vi "LIA Example Host_Backup.vi"() -> ()   [LabVIEW 2017]
uses:
  Program Files (x86)/National Instruments/LabVIEW 2017/examples/Lock-In Amplifier/lib/host/Public/pll settings.ctl
  Program Files (x86)/National Instruments/LabVIEW 2017/examples/Lock-In Amplifier/lib/host/Public/lock-in settings.ctl
  Program Files (x86)/National Instruments/LabVIEW 2017/examples/Lock-In Amplifier/lib/interface/Interface FPGA/LIA Host Interface FPGA.lvclass
  C:/Program Files (x86)/National Instruments/LabVIEW 2017/examples/Lock-In Amplifier/lib/interface/Interface/LIA Host Interface.lvclass
  Program Files (x86)/National Instruments/LabVIEW 2017/examples/Lock-In Amplifier/lib/host/Public/fpga type.ctl
  Program Files (x86)/National Instruments/LabVIEW 2017/examples/Lock-In Amplifier/lib/interface/Interface FPGA/Properties/FpgaSession_GET.vi
  <vilib>/Utility/error.llb/Error Cluster From Error Code.vi
  <vilib>/rvi/errors/niLvFpgaAdjustHostInterfaceError.vi
  <vilib>/rvi/interface/nirviReadWriteControl/nirviReadWriteControl.xnode
  Program Files (x86)/National Instruments/LabVIEW 2017/examples/Lock-In Amplifier/lib/interface/Interface/LIA Host Interface.lvclass
  Program Files (x86)/National Instruments/LabVIEW 2017/examples/Lock-In Amplifier/lib/host/Lock-In Amplifier Example Host.lvlib
  Program Files (x86)/National Instruments/LabVIEW 2017/examples/Lock-In Amplifier/lib/shared/Lock-In Amplifier Example Shared.lvlib
  NiFpgaLv.dll
  <vilib>/rvi/interface/Simulation/niFpgaSimulationCallBeginRW.vi
panel:
  out "pll.q 2":dbl format="%_48p"
  out "pll.vco output 0":fxp<+/-,49,1> format="%#_48g"
  in  "pll.digital config 1":T1={"highLevel"=0.25, "lowLevel"=0.0, "trigger slope"=enum."Positive"}
  in  "pll.digital config 0":T1={"highLevel"=0.25, "lowLevel"=0.0, "trigger slope"=enum."Positive"}
  out "VCO0":dbl[](graph)
  in  "Samples to Read":u32=8000
  out "Result 2":dbl[](graph)=[0.0039863680608536725, 0.0039834652267361085, 0.003976707928082593, 0.003972932599160282, 0.003975670154549236, 0.003979992004370958, 0.003981613977970053, 0.003982100791408192, 0.0039825360403185975, 0.003983392205484175, 0.003985155784781558, 0.003984236112244219, 0.0039802259708269574, 0.003977993518710993, 0.003977332793436194, 0.0039770510070652266, 0.003979204127283512, 0.003981587078878048, 0.003980760652855861, 0.0039774178100061746, 0.0039747546819085605, 0.003975039874942771, 0.003977747825071247, 0.0039813749933174415, 0.003983052660707128, 0.003981864532273667, 0.003980707623093961, 0.003980685672608732, 0.003980632950130394, 0.003980639859174508, 0.003981496097098532, 0.003981835448756967, 0.003981009233135141, 0.003980447530571761, 0.003980017903769632, 0.0039793657225813735, 0.003978886485345096, 0.003978374017005743, 0.003978338111379032, 0.003977708023223816, 0.003974879414400682, 0.0039745951340425896, 0.003978916724054073, 0.003980971523716979, 0.003979875685955788, 0.003980031947639625, 0.003978700378989306, 0.0039759508493841375, 0.003977706550082877, 0.003980981223845854, 0.003980924989904941, 0.00398142250305552, 0.003984342633570469, 0.003985365747847764, 0.003983618653697518, 0.003983156575361657, 0.003984289296932574, 0.003983852105562812, 0.003981528926592434, 0.003979874886696675, 0.003981149393075987, 0.003983128197289955, 0.003982228639004797, 0.003980362051087412, 0.0039805914885188655, 0.003982175398647137, 0.003983227587595888, 0.003982993287403955, 0.003983769026180169, 0.003986244327364255, 0.003986387282293714, 0.003983722992396274, 0.003980432940053473, 0.003977087834015251, 0.003975735503916292, 0.003977729861696195, 0.0039810309668320085, 0.003983694360997393, 0.003985280958577398, 0.003983765419355885, 0.0039787537520719635, 0.003976420955930517, 0.003979177981817055, 0.003980278551671726, 0.003979009157938231, 0.003980564610811761, 0.003982896997404296, 0.003982531965338463, 0.00398162174159325, 0.003981155296610277, 0.003979671906210392, 0.003977937452361379, 0.003976319041318493, 0.0039748268062937105, 0.003975209835147359, 0.0039775478932476726, 0.0039792342447318866, 0.0039792651251529506, 0.003979914577140006, 0.003981608970237078, 0.003981740884947264, 0.003979338128173823, 0.0039772901178909215, 0.003978316936557498, 0.003980306197649136, 0.00398038362175213, 0.003979091211200594, 0.003978807299668593, 0.0039803341878988565, 0.003981042283130753, 0.003979621539503979, 0.003978263643398434, 0.00397885543345211, 0.003980851549467365, 0.003981595814270996, 0.003979534090788055, 0.003976644021712945, 0.0039759454351617, 0.003977357538735612, 0.003978485334334718, 0.003978954978352067, 0.003979752948069682, 0.003980540928132936, 0.003980879798312971, 0.003980939042674783, 0.003981495778424931, 0.0039832350756685946, 0.003984854761938983, 0.003985806865545657, 0.003986168790386302, 0.003983807623814505, 0.003979934662757646, 0.0039786253007486495, 0.0039795163519576555, 0.003980124362455335, 0.0039801733132380475, 0.003981166017222749, 0.003982928364539291, 0.00398290963673646, 0.003980782033860497, 0.0039789779800912676, 0.00397887129554249, 0.003980306008061739, 0.003983353716844369, 0.0039864363131257565, 0.003987887348298469, 0.003988751753916426, 0.003988581162494825, 0.003985527563512181, 0.003981672344151345, 0.003980272419023447, 0.003979888466373754, 0.003978899040399707, 0.003978450628808996, 0.003978327225919375, 0.00397792878270558, 0.003977832419551143, 0.003977741498301615, 0.003977459137679066, 0.003979189237702964, 0.003982949173669057, 0.003983911545934435, 0.003982006472906676, 0.003982384069069882, 0.00398330875633608, 0.003980685479122946, 0.003977745299396019, 0.003978278723887712, 0.0039793920164360235, 0.003978522346022443, 0.003980289178526612, 0.003985997852957612, 0.003988900053516028, 0.003986682772698723, 0.0039831224667016924, 0.003981503976481135, 0.003983123018952358, 0.003985518575956754, 0.003985143703271976, 0.00398195098151325, 0.003980037191873144, 0.003981538653756876, 0.003981542610164564, 0.00397790470261859, 0.003975693240187895, 0.003978387944601431, 0.003982616675137925, 0.003983218136106197, 0.003982211133300878, 0.003982507056608711, 0.003982046262850494, 0.003981635628886928, 0.003982258332005895, 0.003981184985661619, 0.003980668172649484, 0.003984100761381162, 0.003986254732171504, 0.003983367253550932, 0.003980078001556476, 0.003980489638162108, 0.003984508043688629, 0.003988084422329789, 0.003986382148766199, 0.003981484856571877, 0.003978186889057839, 0.003977457434788827, 0.003979266253832761, 0.003982690198689834, 0.003984965342314285, 0.0039834752122414685, 0.003979459150927101, 0.003977443978254645, 0.003978120340943846, 0.003978689408389411, 0.003978751854910974, 0.003979787433988033, 0.003980742378349713, 0.003980678769189533, 0.003982001563511514, 0.003983002537985921, 0.003980921422917653, 0.003978639211764403, 0.0039771230758271735, 0.003976374483646863, 0.003976908953592146, 0.003977079620167436, 0.003977738506023549, 0.003978907819838595, 0.003978870881183955, 0.0039786991463899675, 0.003978616841237893, 0.003977851604700389, 0.003977172646033985, 0.003977513345587875, 0.003978066317637949, 0.00397721868815389, 0.00397542406202231, 0.003973658782307012, 0.00397292656829825, 0.003973899402993055, 0.00397513597871939, 0.003976900361861566, 0.003979478821891459, 0.003980359121710901, 0.0039797019576911785, 0.003979945313537775, 0.003982379006825405, 0.003986819454342757, 0.0039890652386413835, 0.003986060398149026, 0.0039831428691718225, 0.003984496901174192, 0.003986576065894574, 0.003986125938377407, 0.003983891985470712, 0.00398157511744908, 0.00397951127296237, 0.003978500593552686, 0.003979825058149692, 0.003981716302000313, 0.0039817107965979, 0.003980302784099287, 0.003980204028749741, 0.003983014364448184, 0.003984483776541842, 0.003981232134039498, 0.003978395893460694, 0.003978604787843064, 0.003978088591331617, 0.003977643745079901, 0.003981151958603502, 0.003986226271684498, 0.003986688539328525, 0.00398285040357346, 0.003980708004165844, 0.003981031427992134, 0.003980668626391776, 0.003979651616103598, 0.003978880317374354, 0.0039775128160220285, 0.003975690825220382, 0.003977410017621176, 0.003983342449600035, 0.003986190656399481, 0.003983476383350003, 0.003980341993989051, 0.003979157257465969, 0.003978985270725249, 0.003979413120663591, 0.003981198911517176, 0.003983381317756299, 0.003983605961403449, 0.0039822860156277055, 0.003980286417622783, 0.0039768475416357895, 0.0039736879869413134, 0.003972770043621574, 0.003972718526259669, 0.003974519130329869, 0.003978694161036032, 0.003981355840064537, 0.003981296759826837, 0.003979698372206024, 0.003977856657432809, 0.00397795431123421, 0.003979325723467235, 0.003979504894921478, 0.003979619472327822, 0.003981681112522701, 0.003983077441318316, 0.0039811273181025505, 0.003979710446469805, 0.003982873726931343, 0.003985895650077765, 0.003983582096489223, 0.003979810013697831, 0.00397870261963418, 0.003979241406293512, 0.0039797808985378245, 0.003978918139717365, 0.003977535777630392, 0.003977174279037845, 0.003976053026727283, 0.003974360610691553, 0.003975871192530825, 0.00398070376475112, 0.003983714770545892, 0.003981664143647305, 0.003978445706521472, 0.003977845953534627, 0.003977873227033018, 0.003977111770884702, 0.003976355870737198, 0.003975870071358403, 0.003976255642033605, 0.003977987642614486, 0.003980893140634532, 0.003983298672616521, 0.003982542737547836, 0.003980956373361125, 0.003981588316479783, 0.003981099924508738, 0.003979506507396805, 0.003980373061407154, 0.003981050034851546, 0.003979799943130195, 0.00398028280696532, 0.003982919770116164, 0.003984651620736739, 0.003984268351143069, 0.003981935069842658, 0.003979361748262011, 0.003979413820711289, 0.0039819091662637255, 0.003983965670700655, 0.003983195383880426, 0.003979696636904256, 0.003976488408046576, 0.003975787870275286, 0.003978753090618529, 0.003984324294290705, 0.003986722440874599, 0.003984446566004449, 0.003981566760577411, 0.003978855418056195, 0.003977232685187752, 0.003977853017734198, 0.003977827668488712, 0.003977424923808143, 0.0039797462142667165, 0.003983275621354706, 0.003984608790885146, 0.003984263274431654, 0.0039836428598223885, 0.003982289402402122, 0.00398261311929772, 0.003984805689974769, 0.00398377695311104, 0.003979480127359843, 0.003976828270854342, 0.0039763859903618175, 0.003975761395998334, 0.003976091456954722, 0.003979165513275957, 0.003982664353684002, 0.003982886581709554, 0.003980047955028987, 0.0039782590386969975, 0.003980073329210244, 0.003982235704850346, 0.003980773867120832, 0.003977555381209153, 0.003975791737709191, 0.003976838209866267, 0.003980355161348826, 0.003982344986444255, 0.003980347043544887, 0.0039783343900315375, 0.003979105245400305, 0.003979753856154792, 0.0039795020035409, 0.003980682978976577, 0.003983237818856397, 0.003984501894403985, 0.003981990599159561, 0.00397813845175732, 0.0039781783129500805, 0.003981379501095057, 0.003983800319659427, 0.0039857199195843344, 0.003987536828800084, 0.003987384995500621, 0.00398475975584641, 0.003981910972240386, 0.0039812156813270015, 0.003981220039018881, 0.0039801429716929786, 0.003979105844453436, 0.003979900872535141, 0.003981579430532582, 0.003981582347555906, 0.003980139039412083, 0.003978454091171029, 0.003976863715954396, 0.003976033921033562, 0.003977173694941979, 0.003980382420161796, 0.0039840586737615305, 0.0039858618097569475, 0.003984425281235036, 0.003983032946244676, 0.003984565855969025, 0.0039852864498371296, 0.003983009612780214, 0.003981139689177589, 0.0039812527004194544, 0.003981986646524029, 0.003982602846659465, 0.003983280589296684, 0.003983755474126229, 0.0039837132315740445, 0.0039846301134892, 0.003986989494256891, 0.003987488059080713, 0.003983309854404208, 0.0039782076721439665, 0.003976779404301029, 0.0039771905871550045, 0.003977556821407479, 0.003978054614384593, 0.003978322077760754, 0.0039783766773285115, 0.003978026682177368, 0.0039780700494545865, 0.003979334905626531, 0.003980275008436087, 0.003979583910159532, 0.00397806625697346, 0.003977480276853295, 0.003979673909992011, 0.003984152425644857, 0.003986619298023859, 0.003985231117281544, 0.003983500615001195, 0.0039827866633789085, 0.00398137160376901, 0.003980892041843191, 0.003983315682358909, 0.003984865480707667, 0.003983596493280533, 0.003981799731490589, 0.003979158738644041, 0.003977797917050028, 0.003979467394893473, 0.003980100236966837, 0.003979116334303563, 0.003979059817445155, 0.003979986584513668, 0.0039818453133389775, 0.003983893814555208, 0.00398348900651728, 0.003981362260961778, 0.003981989596956523, 0.0039837588119772446, 0.003981791127329015, 0.003979701420423474, 0.003981576725192654, 0.003983063143716834, 0.003982116890878562, 0.003982195467368155, 0.003982486462938863, 0.0039800567872538516, 0.003976082161468444, 0.003974055954040137, 0.003976633941831419, 0.003981412775821396, 0.003983640348413388, 0.003983357995347387, 0.003981415849163097, 0.003977919741453189, 0.003976384895548883, 0.003977484433454275, 0.003977252054023722, 0.0039765150670972235, 0.003978654275285551, 0.003981195762185493, 0.003981712475117914, 0.003981137882798154, 0.00397895360571178, 0.003975775432933715, 0.003975102135976764, 0.0039774497682601925, 0.003978427179725555, 0.003977365226889095, 0.003977594707952847, 0.0039767019639733135, 0.0039727506910756105, 0.0039727350006125706, 0.003978152009208106, 0.003980159374254768, 0.0039778710941888226, 0.003977375595577732, 0.003980037232534828, 0.003983264965478112, 0.003983324524760473, 0.003981049500959955, 0.003980003613294083, 0.003979577212737343, 0.003978403944249703, 0.003977237270009823, 0.003976316160817187, 0.003975980935475114, 0.003977003758017249, 0.003977453398748846, 0.003977510933683602, 0.00398058105512851, 0.0039848047947626366, 0.003986383499902778, 0.003985142716796781, 0.003983150027621312, 0.003983416133046983, 0.003985387313248186, 0.0039844723714048125, 0.003979539219264986, 0.003974621628978131, 0.003973281502577774, 0.0039751541913957454, 0.003977490665905324, 0.003979102054191885, 0.003979381596471701, 0.003977418001187858, 0.003974607390319347, 0.003972382924819207, 0.003971353084165621, 0.003972569948782476, 0.00397516451573597, 0.003976696824166696, 0.003977076730766446, 0.003978236385323944, 0.0039799412673816315, 0.003980671924222786, 0.003980012029596686, 0.003978637131431603, 0.003978993188237805, 0.0039814735245983805, 0.003982739573322356, 0.0039825759490366396, 0.003982518173980329, 0.003981344557208144, 0.003980092358437776, 0.0039806024039760555, 0.00398172681055136, 0.003982319799651587, 0.003981833044348206, 0.003980890395738155, 0.003980723786432255, 0.003980353748032666, 0.003979051107254107, 0.003978363950201649, 0.0039785129216881945, 0.003977883710210291, 0.003975881019731956, 0.003974052048585196, 0.003974685103243776, 0.003977958471936966, 0.003982240156118824, 0.003985098653442519, 0.003984012439980526, 0.003981088700704791, 0.0039804222812716275, 0.003981263262034946, 0.0039822816234043575, 0.003982610443778957, 0.003980656048561382, 0.00397770291899508, 0.003976242147367133, 0.003977345433387912, 0.003979314047879846, 0.003979744798891961, 0.003979349817858955, 0.003979659241239361, 0.0039804007065071135, 0.003980726381835716, 0.003981305356871311, 0.003983663642235815, 0.003987200737890198, 0.0039888053295015526, 0.003986669167392274, 0.003984745900617013, 0.003985989548151111, 0.0039860360759164885, 0.003982841996445306, 0.0039796657749838135, 0.003978478620282327, 0.003979000399240539, 0.003978465766836236, 0.003974640090741505, 0.003971365512208279, 0.003971996504204583, 0.003973775331863526, 0.003975569360546062, 0.003977651962298885, 0.003978271674510117, 0.003977967205246914, 0.00397737164455896, 0.003976686696863666, 0.0039777608428558245, 0.003979548577940783, 0.003980394891505464, 0.003981406684691207, 0.003981515105749858, 0.0039799934957620575, 0.003979236894441649, 0.003978711243243871, 0.003976779191494976, 0.003974763206625327, 0.003973968464875842, 0.003974932132657167, 0.0039789380515777685, 0.003984401295672218, 0.003986189522406129, 0.0039834701725929515, 0.003980876896964074, 0.003981219896273536, 0.00398161832558398, 0.003979026971481225, 0.0039764367788606364, 0.003976914121989127, 0.003978488293238594, 0.003979920584098437, 0.003981391784022643, 0.003981563759137481, 0.0039798070062099285, 0.003978446560805998, 0.003980264683577344, 0.0039827417583317495, 0.003982738530902676, 0.003981310720261693, 0.0039789152179851685, 0.003976986470379223, 0.003977691244145556, 0.0039782020428506416, 0.003976138976957626, 0.003975751526338582, 0.003978975755881895, 0.003981772145538809, 0.00398190266585997, 0.003980256210278689, 0.003978976266084329, 0.003979717924817937, 0.0039820618791054085, 0.003984055133639205, 0.0039842682843533785, 0.003983024743218702, 0.003980806628414367, 0.00397969919132365, 0.0039818567903902044, 0.003984262988199158, 0.003983554601450997, 0.003982491377327015, 0.0039842417870791244, 0.003985864763796289, 0.003984059717472494, 0.003979991963758913, 0.00397622112969835, 0.003975822545353304, 0.003978297051531639, 0.003979084757112439, 0.003979360358689138, 0.00398253720969874, 0.003984459419403273, 0.003981625031530332, 0.003977470787461008, 0.003975547484829462, 0.00397662570312401, 0.003979152537992211, 0.003981564827415988, 0.003983233356038698, 0.003982510000913845, 0.003980070544600705, 0.003977504202257701, 0.003975173437782767, 0.003975389538450331, 0.003977750496773989, 0.003979569013181202, 0.003981351513429408, 0.00398286798035896, 0.003982778257965616, 0.003980372431674904, 0.003976534269270507, 0.003976175306382319, 0.0039803233445810165, 0.00398337679753749, 0.0039834006955887895, 0.003983050335014145, 0.0039823805756204885, 0.003980064467056379, 0.003978699969180845, 0.003980115734287502, 0.003981333010629387, 0.003981386627589539, 0.003982395720148015, 0.003984079152264324, 0.003985038171922114, 0.003985167413950783, 0.003983941807828037, 0.003982038483599197, 0.003980884988355782, 0.003979008103024772, 0.003976990229437761, 0.003977162586203987, 0.003976899320749507, 0.003974284450258375, 0.0039720946084108285, 0.003972026230624667, 0.00397374886027822, 0.003976367439575529, 0.003977842425566234, 0.003977093338184401, 0.003976103952084634, 0.0039763017689312865, 0.003976092417151285, 0.003975060626111278, 0.003975065135869968, 0.0039763107365488526, 0.003977352867079649, 0.003977969349847659, 0.003978553095446936, 0.003979036478021424, 0.003978983042730239, 0.003978741465652077, 0.003979340578042503, 0.003979701242850902, 0.003978430882799382, 0.003976652233153723, 0.0039765179596725, 0.00397795735513347, 0.003979565201195335, 0.003981345484242718, 0.003981469312432307, 0.003978889562823616, 0.003976624913683742, 0.0039761610778784534, 0.003977824959453653, 0.00398214069195037, 0.00398742195165944, 0.0039896995458981776, 0.003986037631195687, 0.003979967695862646, 0.003977040393717214, 0.003977674391227534, 0.0039792757272066395, 0.003979552641289948, 0.003978935698737408, 0.003978281367870273, 0.003977642996036234, 0.003978731377392299, 0.003981539171295274, 0.003984238656581007, 0.003985224180818125, 0.003983057443176566, 0.003979499397401518, 0.003978410752375987, 0.003979776671656836, 0.003980391436479124, 0.003980049271568817, 0.003980241632899643, 0.003980339940009103, 0.0039807557540897055, 0.0039822609635872695, 0.003983176627180919, 0.003983926928775935, 0.003985551548307111, 0.003985646813215484, 0.003983680363220629, 0.003982849003454181, 0.003985561835201112, 0.003988929187930998, 0.003987829703049252, 0.003983503133059348, 0.003980623127040725, 0.003981481278276747, 0.003984305894978182, 0.003983197724472904, 0.003977985889312162, 0.003974146671127731, 0.003972623406271078, 0.0039726346931309026, 0.003974042725941328, 0.003976747169016437, 0.003981487948263495, 0.00398504490845982, 0.003983113583811858, 0.003978458043433113, 0.003976326104421417, 0.003977793620755946, 0.003980780035179106, 0.003981852492902647, 0.0039806181319497844, 0.003979685704064992, 0.0039783801316026325, 0.003976448851123849, 0.003976660341366401, 0.003978477345490919, 0.003980078187884992, 0.0039818262398588124, 0.003983429147918595, 0.003984344934371185, 0.00398413317542814, 0.003982099362293185, 0.003979385893110493, 0.00397997889618068, 0.0039846267580415816, 0.0039861289961856386, 0.003981209101616648, 0.003976602731196693, 0.003975722568327848, 0.0039750119685239855, 0.003974583143683917, 0.003977236560717556, 0.003982154517706716, 0.003986351620900945, 0.0039867699783994685, 0.003983698012302503, 0.003979936072057596, 0.003977518007059206, 0.003977251859838127, 0.003977404443913313, 0.003977064129850515, 0.0039774177115842945, 0.003978840238485831, 0.003981328955739816, 0.003983214287842484, 0.003982316329195417, 0.003979705808360979, 0.003978095353210538, 0.0039780303866684755, 0.003977773027807622, 0.003976670088152897, 0.0039760803031386625, 0.003977074375590223, 0.0039785954201575924, 0.00397900504669715, 0.003978684455654764, 0.003979150345052722, 0.003980073213741131, 0.00397922400508169, 0.003976634199148333, 0.003973792948548973, 0.003971947735484429, 0.003973449300176407, 0.003977365527006807, 0.003979173865527555, 0.003978565338237246, 0.003979438592656055, 0.003982226081643567, 0.003984568899889969, 0.003985383545762023, 0.00398379361244337, 0.003980766058359194, 0.0039789937389582706, 0.003978725628367393, 0.003978486455318838, 0.00397930624856685, 0.003983076144599588, 0.003986916500922116, 0.003987391456195043, 0.003985187981902368, 0.0039814220323227505, 0.0039782599038656885, 0.0039793530195430405, 0.0039836665900997974, 0.003985418628529121, 0.003983107447318631, 0.0039807533716833795, 0.003980452673891609, 0.00398121246321292, 0.003981579245847072, 0.0039806453902812115, 0.0039793147147476815, 0.003977426450764091, 0.003974647202875613, 0.003975534272025265, 0.003980944354864695, 0.0039837113287362075, 0.00398066195437423, 0.003976075275215913, 0.003973624263519756, 0.003972642118978977, 0.0039721981348636755, 0.003972418027957137, 0.003973516751950605, 0.003975424914188026, 0.0039764420265992395, 0.003976805487305147, 0.003977527309148269, 0.003977276759045344, 0.003977874650012254, 0.003981908131747179, 0.003985791593126928, 0.003987332531377609, 0.003988917999303813, 0.0039898000436693675, 0.003988775524159052, 0.003986804137343182, 0.003983974012608901, 0.003981762439486124, 0.0039812892508868285, 0.003981024159819735, 0.0039812211576087195, 0.00398236019474162, 0.003983547327636211, 0.003984231855020959, 0.003982225962846631, 0.0039783147688324414, 0.003977077736042259, 0.0039784658388757775, 0.003979775888746237, 0.003979987933157361, 0.003979458851215214, 0.0039793476299291725, 0.003978612550414, 0.003976314387840179, 0.003975056548604429, 0.003977366661085867, 0.003981128734793488, 0.003982649122544232, 0.003982768691437142, 0.003982005871057322, 0.003980190872963164, 0.0039813036494263454, 0.003984124532118742, 0.003982475946791014, 0.003977761415616033, 0.003974659343488677, 0.003972846843811938, 0.003972806715625865, 0.003975651569164522, 0.003977963611383471, 0.003977873468104301, 0.003978068385375542, 0.003979488335530391, 0.003979110480443132, 0.003977206961489088, 0.0039789202289513695, 0.003983288863755289, 0.003984077121378504, 0.0039822076981657125, 0.003981856479113935, 0.00398181012214159, 0.003980737648898447, 0.003980066845379656, 0.003978715861692618, 0.0039758546373015995, 0.003975257761946412, 0.003977846923118978, 0.003980669832971535, 0.003982954669011326, 0.0039835557510074, 0.003981614603206939, 0.003980593956608991, 0.0039822666237705985, 0.003982790656945957, 0.00398006863105295, 0.003977102352752207, 0.003976331524483975, 0.003976025112422648, 0.003975993713770331, 0.003978360261045454, 0.003980515957965241, 0.003980492262176662, 0.0039803134217181214, 0.003981116190908811, 0.003983517947269706, 0.003984911931008131, 0.0039824874179596684, 0.003979324028877534, 0.003976903166459353, 0.003973952933671413, 0.003972768156739406, 0.003974518699813129, 0.003977092525553969, 0.003979000361980179, 0.003979473587682066, 0.00397880296134308, 0.0039773501151807765, 0.003975775190348078, 0.003976784857872222, 0.003980497553940501, 0.003982816679431947, 0.003982101922554104, 0.00398090377027712, 0.003980526960595199, 0.003980273848589513, 0.00398004016560462, 0.0039796316262196724, 0.003978590884515269, 0.003977695523808001, 0.003978113283674883, 0.003978093677450509, 0.003976234690895188, 0.003975571953397801, 0.003977429275899129, 0.003979690179076107, 0.003981314699049087, 0.003982365023104846, 0.00398219328738418, 0.003979413083539485, 0.003976093378332462, 0.003977107605273904, 0.003981169964969415, 0.003983559556918537, 0.003983587714059575, 0.003981431842795316, 0.003978969249534734, 0.003978935715453941, 0.003980895947219992, 0.003982877361418654, 0.003982597564966746, 0.003980748884707083, 0.003980175712387027, 0.003981130286463459, 0.003980398082433253, 0.003977314767296546, 0.003978106092339979, 0.003983020800341056, 0.003984163473727247, 0.003981822309170868, 0.00398186832723127, 0.003983498351935705, 0.003982833932537083, 0.00397963340189174, 0.003976943389420637, 0.003977245664763129, 0.003979882345903582, 0.003982544930166112, 0.003982603116630313, 0.003980387169699541, 0.003978424228600121, 0.003976559770536161, 0.003975981643434425, 0.003978714956440631, 0.0039812885056061615, 0.003980169419182908, 0.003978061693649715, 0.003979346532064259, 0.0039829775933541214, 0.003983549530300931, 0.003980744676411625, 0.003979164800276976, 0.003980084512057897, 0.003981743527813305, 0.003982186814042334, 0.003981262059743135, 0.003980155795563241, 0.0039791162400227426, 0.003978750075723301, 0.003979895399989306, 0.003982175444757632, 0.0039839269838620696, 0.003982767707209037, 0.003979702364871831, 0.0039794049219338224, 0.0039808389302070256, 0.003979538938519838, 0.003977892739263718, 0.0039786753680560085, 0.003979574852086779, 0.003979358746771128, 0.003978307718653613, 0.003977615907680387, 0.003980297680133449, 0.00398455438897639, 0.003985124482927759, 0.0039830989248438795, 0.0039821580726706815, 0.003983029891208001, 0.003985361124408492, 0.003986676078649965, 0.003985371613000642, 0.003984264122271375, 0.003985115332201757, 0.003985380850084425, 0.003984091577875379, 0.00398348442375365, 0.003982335908804991, 0.003979130290729062, 0.0039765271382101374, 0.003975761283694023, 0.003977309789773401, 0.003980495824565586, 0.003982011694418642, 0.003982418786917205, 0.003983446588687851, 0.003983373050037224, 0.003981312358611243, 0.003979194733814413, 0.003978205677460493, 0.0039771896308695015, 0.0039760863754637644, 0.0039754517556096595, 0.003975021126421098, 0.0039743248319844705, 0.003974288300301103, 0.003976760901184927, 0.003978623824061758, 0.003977594513440992, 0.003978555080478624, 0.0039821930546257, 0.003983594593330003, 0.003982405089531026, 0.003981856594388102, 0.003982187387509669, 0.003981223313549715, 0.0039807403298629356, 0.003983347548875419, 0.00398522027841444, 0.003983423163518952, 0.003980738682966747, 0.003979015525778642, 0.00397895173097921, 0.0039793029748609295, 0.003977636235713472, 0.0039759450751720654, 0.003976485471559254, 0.003977655809397979, 0.003977429349678956, 0.003977993254621377, 0.003981879567469959, 0.003985239298407153, 0.003983416989748803, 0.003979679076637758, 0.003980365788350991, 0.00398253381694978, 0.003981285993316625, 0.003979848440676178, 0.003980921832108509, 0.003982172952809117, 0.003981158711881339, 0.0039800950644021515, 0.00398118948495695, 0.0039812176124992054, 0.003979616502188085, 0.003979039178311631, 0.003977916218000592, 0.003975378585060592, 0.003973131227205391, 0.003971918687654648, 0.0039734481724517925, 0.003976717516063116, 0.003977014875929817, 0.003973625298260909, 0.00397052208057938, 0.003971026897799082, 0.00397378807698498, 0.003973657752896502, 0.003971306556533753, 0.003973085672003789, 0.0039772575872008996, 0.003979194823547542, 0.003980317158812024, 0.003981292049856421, 0.0039831232472903105, 0.003987251711291331, 0.003989738525540101, 0.003987456983345958, 0.003984035239048443, 0.003981801724854245, 0.003979640732521801, 0.003978737305790658, 0.0039786476741947826, 0.00397791462118473, 0.0039777749317880026, 0.003978196073117516, 0.003978760709114377, 0.003979171876865028, 0.00397890829124455, 0.003979693827835825, 0.003982373595558498, 0.003984460873171954, 0.003983641771434025, 0.003980399820629003, 0.003977143685017755, 0.003976739331852892, 0.003978646828280886, 0.003979812280227829, 0.003981210448487633, 0.003983015756720717, 0.0039817333859492165, 0.003979002376219683, 0.003979107817471822, 0.003981211465274229, 0.003982606424709189, 0.0039832693787421585, 0.003983051654033211, 0.003979894748497823, 0.003975385528241426, 0.003973522960580348, 0.003974656401160778, 0.003978349370676319, 0.003982892688988913, 0.003983594701533446, 0.003981272021551873, 0.00398141035625862, 0.003984034138904719, 0.003986270231203048, 0.003987371878162886, 0.003985805363107296, 0.0039817409828335005, 0.0039800045857511165, 0.003982567734983381, 0.003985107690832858, 0.003984026682255706, 0.003981247498766315, 0.003979945374079749, 0.0039792207502099, 0.0039776515097977305, 0.003977553621094195, 0.003979640591280083, 0.003979802663149316, 0.003977016451329748, 0.003975536826100867, 0.0039779635670275015, 0.0039826413914955915, 0.003984064601877063, 0.003980053006106213, 0.003976825452021229, 0.003978578253056492, 0.003981962351984016, 0.003982619824916695, 0.003981592297708066, 0.003982013868026151, 0.003982298477104434, 0.003980510565228737, 0.003977882740497247, 0.003975967656348129, 0.003974813724179058, 0.00397367248316158, 0.003973745754006388, 0.0039765977484971975, 0.0039808396448549836, 0.003983537135687354, 0.003982979750045097, 0.0039799912584952395, 0.003977658737727139, 0.003977733078746502, 0.003978891204631039, 0.003979577122098112, 0.003978841805351333, 0.003976426768058204, 0.003974922818355137, 0.003977647373739251, 0.003981615548013295, 0.003980917845452167, 0.003977078549640621, 0.00397536837004931, 0.0039759780432128385, 0.0039762392964120645, 0.003976725341889077, 0.003978542997694838, 0.003979204759203014, 0.003978218625753375, 0.003978442388650503, 0.0039788453982813115, 0.003977975565517368, 0.003980073457269644, 0.003984761099604855, 0.003984821629434982, 0.003979963390238673, 0.003976945779116363, 0.003978204691117046, 0.003979426407224877, 0.003978475158178936, 0.003978531771511002, 0.003979999568456761, 0.003980753652738751, 0.003982165401077395, 0.003984447066973862, 0.003984125648018166, 0.003981421270245027, 0.003980137096143932, 0.003981451103728136, 0.003982679633245892, 0.003982258706786912, 0.003981488736817787, 0.003980199736889629, 0.003979185774484476, 0.003980638280255229, 0.003983363518089745, 0.003983860950202896, 0.003981813894202404, 0.00398042291412263, 0.003979831315147897, 0.003979837933985523, 0.003981936562422305, 0.003983040777982667, 0.00398078405540393, 0.003978119547563092, 0.003977041795773243, 0.003977311074221384, 0.003978894939935517, 0.003981016940009896, 0.003981602804992968, 0.003980790460175742, 0.003980832038069681, 0.003980246643918975, 0.0039769227718498, 0.003974138089899075, 0.003975488971503561, 0.003979858248285364, 0.003982834257554093, 0.003982224164074203, 0.003980711646259053, 0.003980044834544112, 0.003980217296298432, 0.0039817160981850605, 0.003983443484275833, 0.00398371428718893, 0.003982610604973739, 0.003981524871862345, 0.003980620390250896, 0.003980108148874865, 0.003980783373574936, 0.003982060412047107, 0.003983948662640071, 0.003986074427056052, 0.0039863962532675, 0.003985134297653663, 0.003985193406920106, 0.003985882297205966, 0.00398405309546629, 0.003982542021274245, 0.003983904862923795, 0.003983049463213574, 0.003978382592098956, 0.003975436268357411, 0.003976550738406553, 0.003978588341625853, 0.003978228638552719, 0.003976405440297321, 0.003976619742890873, 0.003978250186032161, 0.003978039025728405, 0.003977476248553813, 0.003979160885704842, 0.003981493321230651, 0.003982737572559862, 0.003982199226558208, 0.0039800803582359014, 0.003978621713377863, 0.0039789827585751045, 0.003980856722724818, 0.003982756548377972, 0.003982152493373126, 0.003980001403718744, 0.003977809718787921, 0.003974775668880134, 0.003972822966618998, 0.003974116674563762, 0.0039774266158550745, 0.00398013621130506, 0.0039805969751882725, 0.003980839984234072, 0.003981913158604893, 0.0039809020006479, 0.003978043639507173, 0.0039761023336582525, 0.003975735479197253, 0.003977237164066012, 0.003979156890400347, 0.003977959631900995, 0.003975664541786072, 0.003977015948163484, 0.003979800747511443, 0.00398036358261194, 0.0039791333003214744, 0.003977584037880255, 0.003977903249913146, 0.003980824679784317, 0.003982139767034596, 0.003979923660558457, 0.003979679130910815, 0.003982887698775242, 0.0039839573368327, 0.003981415865620109, 0.003980026959041138, 0.0039826530815789355, 0.003985032531173712, 0.003983170211885002, 0.003981229208051504, 0.0039831419107672975, 0.003985314929199347, 0.003984736539562992, 0.003982047625534495, 0.003978092253258514, 0.003976171860381736, 0.003977097600080971, 0.003976715465265732, 0.003975528628593147, 0.003976225728987328, 0.003976577835919223, 0.003976080688442137, 0.003977065463732254, 0.003979095970022937, 0.003980869775893732, 0.003980031320668816, 0.003976488044518928, 0.003976033855949846, 0.003980667305431748, 0.0039852116356552105, 0.0039850375694942325, 0.003981444890417225, 0.003979055176481802, 0.003979334454276697, 0.003981964690537828, 0.003985277726719733, 0.003985372395858868, 0.0039828274764985615, 0.00398149899661329, 0.003982572698372539, 0.003983587744335812, 0.0039811751383610535, 0.003978667166125552, 0.0039799350381902725, 0.003980131396301726, 0.00397701659831602, 0.003976251438084941, 0.003980000546690863, 0.003984326491579235, 0.003985406726219048, 0.0039823257385474325, 0.003978328034980272, 0.0039781141261135775, 0.0039825817773765605, 0.003987019086670008, 0.003986378504586017, 0.003982321435581621, 0.003979287104622096, 0.003978757690781972, 0.003979867479212055, 0.003980990323479186, 0.003981524507956091, 0.003980930294299735, 0.003979714774223713, 0.0039798609378699, 0.003980489633458653, 0.003980954515594047, 0.003982451454848569, 0.003983592354646729, 0.003983023643667566, 0.003981780453426345, 0.003980150677261656, 0.003977939858915903, 0.003976663953581718, 0.003976567267764581, 0.003976742276555209, 0.003977026113949605, 0.0039759017010204374, 0.003974620894287012, 0.003976550878632898, 0.0039794254344922226, 0.003980053670982793, 0.003978893617156679, 0.003976881683576605, 0.00397681165987789, 0.003980650125893448, 0.0039839316298084905, 0.003981472200463117, 0.0039760224680521015, 0.0039749080711558235, 0.003978573498169757, 0.003980834012888352, 0.003980277146134611, 0.0039798290866767646, 0.003979696358708986, 0.003979243706929482, 0.003979458656012906, 0.003980735616066876, 0.003981573829207304, 0.003981333949018392, 0.003980334275621537, 0.003979296577206264, 0.00398092191490291, 0.003984615251211943, 0.003986054489476058, 0.003984084777022521, 0.003980669260339174, 0.003977687646522303, 0.00397633130425075, 0.003976487048231085, 0.003975980482120383, 0.00397444740535783, 0.003974517679956067, 0.003976443223808739, 0.003978538570867421, 0.003978807200209765, 0.003977011707770822, 0.003976664972314686, 0.003978300482415657, 0.003979540018477265, 0.003980498057458205, 0.0039823678050551255, 0.00398426523072378, 0.0039835282605164635, 0.003981308831879845, 0.0039816179762867, 0.0039839099042353575, 0.003986082753664326, 0.003988042873930375, 0.003987392251139272, 0.0039838210259798895, 0.00398181843022356, 0.003983219826813076, 0.00398609138070574, 0.003986520539064208, 0.003982348342074492, 0.003977350315412907, 0.003974825714130103, 0.003975001827794674, 0.003977881508835268, 0.00397983876716173, 0.003978133890651639, 0.003976987943834461, 0.003979209753329046, 0.003981358977343799, 0.0039804571205447345, 0.003978705675329452, 0.0039804624250637495, 0.0039837235542263625, 0.003982785445988357, 0.003979053783229923, 0.003977419940931196, 0.003979800732348097, 0.003984036663505942, 0.003984974435885952, 0.003981722544176443, 0.003978600948416513, 0.003978002716351739, 0.003978319099118849, 0.003977869650191021, 0.003977770879884532, 0.003979235856318206, 0.003980787554768288, 0.003981054721549102, 0.003981475992411021, 0.003983322700911616, 0.00398459773304639, 0.003983058390335627, 0.0039794076200789594, 0.003977001169472031, 0.00397933347944537, 0.0039834383415941034, 0.003981871562804738, 0.003976686265121069, 0.003976457926069695, 0.003980452398060831, 0.003982842756804102, 0.003983116591155044, 0.003983704020879471, 0.003986445190217968, 0.00398909119912337, 0.003987010336441944, 0.003983414412622325, 0.003984104843046473, 0.00398551784454822, 0.003983372321284873, 0.00398108339487192, 0.003981720491102667, 0.00398191641173596, 0.003978647712721205, 0.003975995437829183, 0.003977792287636826, 0.003980350600781975, 0.003980040640280543, 0.00397852709799242, 0.003976632207578901, 0.0039753732216189636, 0.003976682038481194, 0.003978276072790252, 0.003979894658056205, 0.003982765760135251, 0.003983833023602612, 0.003981797166506561, 0.00397954894130544, 0.003980166421746046, 0.00398235147254963, 0.003982998746410941, 0.0039811285591011755, 0.003977696908878916, 0.003977118739538499, 0.00398008944064117, 0.003981482740950911, 0.003979930882977621, 0.00397743087136605, 0.003975971252553409, 0.003977462863057397, 0.003980674791534549, 0.003982380782257275, 0.003981526409016917, 0.003980107334962722, 0.003981167294126887, 0.003983703414652771, 0.00398420490645264, 0.003982791413991762, 0.003981005836849114, 0.003978678257854902, 0.003976499847155555, 0.003977437797218255, 0.003980424883737011, 0.003980326027344289, 0.003979196440516551, 0.003980845589105199, 0.003981763032187864, 0.003981054495160551, 0.003981235591409589, 0.003980451669450776, 0.0039773865429069254, 0.00397561327819297, 0.003977100584558286, 0.003979076444861173, 0.003980297135872896, 0.003981822553022909, 0.003982609342912283, 0.003980864418373111, 0.003978282057316814, 0.003978422281035807, 0.003979783907547497, 0.0039792569116670826, 0.003979812051897325, 0.003983690847610773, 0.003986505256641431, 0.003984122438926664, 0.00397960450003522, 0.003979069664485006, 0.003981195343956562, 0.003981997230810312, 0.0039832777628919565, 0.003984922802692337, 0.003984097756897918, 0.003982506835353294, 0.00398276576533815, 0.003983780947940771, 0.003983491783514083, 0.003982192919674611, 0.003981049887130392, 0.0039795336732412175, 0.0039780498454925015, 0.0039777558937685465, 0.00397875942314283, 0.003980791462300775, 0.003980644242681716, 0.003978019770326027, 0.00397838840741479, 0.003981094641202824, 0.003981527119447348, 0.003981231781193979, 0.003982419751017016, 0.003982893388840162, 0.0039811587589446305, 0.003979287914954477, 0.003979705406330276, 0.003982313348835465, 0.003984826699072945, 0.003984560228902292, 0.00398044421241466, 0.003975828438144637, 0.0039749358705011995, 0.003976215290702679, 0.003976569770132877, 0.003975021779170308, 0.003972964919774096, 0.003974294532385254, 0.003976839604263706, 0.0039759723311441186, 0.003974834950478125, 0.003976394430271158, 0.003978875799636114, 0.003980345412888455, 0.003981232956825354, 0.003983301174181986, 0.003985089864527834, 0.003983816948260292, 0.003981233980028774, 0.003980784024137563, 0.0039824962565403, 0.003983963328384499, 0.003981997324169284, 0.003978207187765573, 0.003978196951401253, 0.0039819972264322516, 0.00398557328750668, 0.003986746679901954, 0.0039860697379306385, 0.003984758252749328, 0.003982565355105981, 0.0039794010173368945, 0.003977517617529265, 0.0039789565045569185, 0.003980415474610019, 0.0039783577960271115, 0.003976203600247609, 0.0039770700956976955, 0.0039796760325666565, 0.003981992186612386, 0.003981618979916626, 0.003979073354562346, 0.003977135626932566, 0.00397603671184648, 0.003976420834526046, 0.003978215005732462, 0.003978158631138276, 0.003977620674882885, 0.003979524105166559, 0.003980073864498317, 0.003976732087475557, 0.003973440587860436, 0.003973740795186001, 0.003977420410965805, 0.003981581319918532, 0.003982947445088291, 0.003982018405176985, 0.003979936339929113, 0.003976765570600322, 0.003975307664693699, 0.00397717628337053, 0.003980538350126554, 0.003983565227955119, 0.003985093324970469, 0.003985346114652908, 0.0039851769858805, 0.003983111123840236, 0.003979416204281513, 0.003978754784272771, 0.003982152441837931, 0.003984552447743194, 0.003983350784890174, 0.003981413511676224, 0.003980441089932959, 0.003978644299059765, 0.003976625703574787, 0.003976937703597712, 0.003978018628758417, 0.003978153061952123, 0.003978612110596774, 0.003979410621509879, 0.003980344936763674, 0.003981399327838175, 0.003980511915169716, 0.0039782594955080795, 0.003978898117406929, 0.0039808393749142384, 0.003980369130952465, 0.003980494255639036, 0.003982458340161773, 0.003983322410304637, 0.003982200837774065, 0.003980923638073811, 0.0039821856113854345, 0.003985516151544953, 0.003987504781818696, 0.00398639201384877, 0.003983520994705897, 0.00398210342383452, 0.003983097872455665, 0.0039833503902948824, 0.003980826669473829, 0.003977383722986291, 0.003975952411614413, 0.0039765473225302625, 0.0039784950700595045, 0.00398178294276151, 0.003982087151434271, 0.003979264120615359, 0.0039800288740998585, 0.003984740946969013, 0.003987583380635075, 0.0039848324786377785, 0.003979336323058747, 0.003977017510941184, 0.003978459215879899, 0.003980154439026382, 0.003981467435214172, 0.003982944961763137, 0.003982254383022156, 0.003979933868386716, 0.003980160298696735, 0.003982485896065806, 0.00398346197794012, 0.0039823797109441, 0.003980532523050853, 0.003979688916405943, 0.00398076954813637, 0.0039826642343657025, 0.003982786486702663, 0.003980180868902629, 0.0039778557841841, 0.003979284790976656, 0.003983799275513648, 0.0039869668002875495, 0.003985270774969235, 0.003981669950420741, 0.003981159113970482, 0.003983252358314593, 0.003985254217573198, 0.003985416441331974, 0.003983203154028067, 0.003980034997262223, 0.003979101719660604, 0.003980798247778421, 0.003980184602307087, 0.00397666728941187, 0.003975980095220212, 0.0039786014322548136, 0.003979601159884406, 0.00397862452850414, 0.003978886889883609, 0.003979152242347788, 0.003976596530977417, 0.0039738470034338105, 0.003974707135773609, 0.003976726842203554, 0.003975435206138856, 0.003973227802032742, 0.003975388709941386, 0.003981562317343599, 0.003987427186256705, 0.003989726636335336, 0.003987802190259164, 0.003983347020890189, 0.003979742561774817, 0.003978273940531642, 0.003978030365195505, 0.003979166776045112, 0.003980136483166431, 0.003979092728439485, 0.0039772354500607005, 0.0039755792359054305, 0.003974479041064347, 0.003975111617170037, 0.003977291150669083, 0.003978825680661359, 0.00397996245572211, 0.00398227162380318, 0.003984647832750007, 0.003986284670137607, 0.003986697328944248, 0.003985417521417754, 0.0039839346334049775, 0.00398347555043011, 0.003983205930136137, 0.00398070235203716, 0.003976748974812923, 0.003975233423234118, 0.003976544293385957, 0.003979193419383836, 0.003981870777837675, 0.003983088370781337, 0.003983188202260073, 0.003982761337973724, 0.003980832388996442, 0.003977494954797085, 0.003975230167199459, 0.0039750156759105135, 0.003974965041093329, 0.003975553606117713, 0.003977929245430073, 0.0039790159127192784, 0.003978141073576601, 0.003977861314810282, 0.003977842887149551, 0.0039775401044030365, 0.003977529124982839, 0.00397733840907286, 0.003977300190341391, 0.003978316464437354, 0.003978741774444075, 0.003977333514756551, 0.003976051242313199, 0.003976463891249626, 0.003979051301113224, 0.003982587746143712, 0.003983767095214161, 0.003982878095068564, 0.00398231244237889, 0.003981470942921979, 0.003980718822575232, 0.003981264742134407, 0.003981083402365196, 0.003979617923778215, 0.003979079934982027, 0.003978612166737189, 0.003976697390197674, 0.00397537713925854, 0.0039756809402528796, 0.003976807013215364, 0.003978035185188689, 0.003976603997993078, 0.003972405090856017, 0.003970968907838601, 0.003974655491417799, 0.0039778248200223, 0.003976569365212407, 0.003974905469759597, 0.003976766750882373, 0.003981383485380135, 0.00398432853854629, 0.003982506464076941, 0.003978702948704632, 0.003976413718171325, 0.003976908300555339, 0.003979234065943796, 0.003979332831016226, 0.003975733674159248, 0.003972947093051985, 0.0039744904149888695, 0.003978758726346908, 0.003982641138560387, 0.003983725107684731, 0.003981709291406732, 0.003978917113292253, 0.003977104215637433, 0.0039765317930494665, 0.003977268187779722, 0.003978577162569696, 0.003980160172414112, 0.003982024574796909, 0.003981492819084455, 0.003978141370665758, 0.003975254080400424, 0.003974619747690328, 0.0039776515271878355, 0.003981986302415632, 0.003982934257307543, 0.003981870554930871, 0.003982104296708313, 0.0039847097461042265, 0.003988132729987256, 0.0039888279650053425, 0.003987015495068171, 0.003984679479035331, 0.003981257369583279, 0.00397768195465082, 0.0039767898864814695, 0.0039796114158642095, 0.003984185210966746, 0.003986327741798733, 0.003984893017648091, 0.0039828401293103095, 0.003981338061149414, 0.003979070384647841, 0.003976923268061201, 0.00397828379918129, 0.00398141041118076, 0.003981508945655101, 0.003980910588486213, 0.003981911978365021, 0.003981530653317517, 0.003980719902025504, 0.003981210245567557, 0.00398021711464625, 0.003977178053121612, 0.003976404508326288, 0.003979956311781098, 0.003982270518685749, 0.003980239402988643, 0.003979180024550727, 0.0039800965753906134, 0.003979546297551935, 0.003979575085543971, 0.003981713953566729, 0.003983588775941205, 0.0039855942171031665, 0.003987028924608211, 0.003983659736349213, 0.003977593271757678, 0.0039751855027903415, 0.003977441392311144, 0.003980564015485558, 0.003982007356590616, 0.003983181463094195, 0.003983779144265405, 0.003982869864763861, 0.003981719330332108, 0.003979686308300706, 0.0039777655663639725, 0.003977463794452425, 0.003975925016051441, 0.003972672482849184, 0.0039711331876262496, 0.003972696828325609, 0.003976784050061718, 0.003980743768737575, 0.0039806327390801465, 0.003977402952918321, 0.003975547097828529, 0.003976323470220061, 0.003978299245303643, 0.003980523675770113, 0.003982981354025069, 0.003984758427777584, 0.00398534270943657, 0.003986537436464047, 0.003987195731455987, 0.003983999652486442, 0.003979213899319078, 0.003977625156442222, 0.003978192249860361, 0.003978329383507582, 0.003980148749083131, 0.003982575296372368, 0.003981570162043734, 0.003980377771675154, 0.0039823385670842695, 0.003983904932702141, 0.00398353741704041, 0.0039823574487762685, 0.003980149025360017, 0.003978436496680693, 0.003978440740042261, 0.003979217846675801, 0.003981258796273241, 0.003984180886428258, 0.003984287841128788, 0.003981885227684841, 0.003982468210707445, 0.003986012356272324, 0.003986870336495815, 0.003984872536461842]
  out "Waveform Graph":cluster{"f0":dbl, "df":dbl, "magnitude":dbl[]}[](graph)=[{"f0"=0.0, "df"=48828.125, "magnitude"=[-46.93833321413425, -48.890085398745086, -57.05864793570993, -63.948010145782, -57.10808944274945, -63.55723661730865, -57.477633254873524, -63.388970771981256, -57.83858653215573, -63.04278294236552, -58.310732731480286, -62.75659424633111, -59.01913953160205, -62.55034509450798, -59.76806715246457, -62.45290461669743, -60.67593939903783, -62.55360847730091, -61.80337052022501, -62.7503089432639, -62.95874542404657, -63.17666796807587, -64.24815178765463, -63.58179265883102, -65.96263589732504, -64.29834519828907, -67.76706631207706, -65.25530419899528, -69.69720964445415, -66.48978075872667, -72.0836829037614, -67.87758710008302, -74.95546090477261, -70.02468767091023, -78.46318325872932, -72.61789596314395, -82.74302220692796, -76.45363219872509, -86.93156331597662, -81.93411626073177, -89.39593580415576, -99.6170681323641, -88.66324403386615, -83.63767905833946, -86.78510178329685, -77.97514394138707, -83.83057336078254, -74.91042135055551, -81.5475507560879, -73.50059696206921, -78.86254697144325, -72.13420582514291, -77.68352683311363, -71.47125092202423, -75.95623700109, -71.27989762649543, -74.95441595981052, -71.25879209888319, -73.9595113284693, -71.56173669996721, -73.54477863881124, -72.29773534656574, -73.22367389861854, -72.96381308648769, -72.9988078797969, -73.86835428297962, -72.95305526553327, -75.2471462028992, -73.52456103236882, -76.90120154185578, -74.35415308379046, -78.75438807181995, -75.52159448517878, -81.97850502570516, -77.0522962144752, -83.72534671678167, -79.22667312669566, -87.72245228429632, -82.41997364153613, -92.98958808340201, -88.94092629488937, -99.50542487601304, -104.43928510750062, -96.68595945743522, -89.84335052432984, -91.19624554856414, -83.82262417189582, -90.01723416008254, -80.15754604679948, -85.81708298956508, -78.30065773404802, -85.06593198935606, -77.23628138343811, -82.71304646807387, -76.35856258445034, -81.61855339489769, -75.96594028137565, -80.15275231432624, -75.79741810419392, -78.97129025392613, -75.86427195094097, -78.17458456209165, -76.12085849656066, -77.85383262432903, -76.74912507995519, -77.25671541218556, -77.8982284228998, -77.8212535613011, -78.99364420828655, -77.9535986594113, -80.5765883437286, -78.71247862445587, -82.81330063919576, -79.90075393045993, -84.51582581828501, -80.84734822816016, -88.15097620058117, -83.06948686637503, -90.43795841683013, -87.05804894598725, -100.9044462888944, -91.16184483511006, -99.25318703849094, -113.00302254650566, -101.23938945826266, -94.74360211928621, -93.60935601063579, -86.60563663892235, -90.06499901122993, -82.85388280403822, -89.22123700503676, -81.17742163079215, -87.46988992571065, -80.0064748842741, -85.67242615027025, -79.5534829705813, -85.2386741467478, -78.36875630953557, -83.74067249570277, -78.58966459550572, -82.65136916700945, -78.45793002426842, -81.60291278830285, -78.78545275144468, -81.44873599291637, -79.46689782726857, -80.9546312968039, -80.34286350947234, -80.64680657897753, -81.40467594015718, -81.45416553874705, -82.91913176326895, -82.01356243362385, -84.4698494074905, -82.43677736126503, -86.83038860613686, -84.19971850756579, -89.09446672366998, -85.50637044704303, -93.27140345100959, -90.41560771649186, -102.15908510562295, -94.5879404286508, -103.56313351942903, -113.25509523061405, -96.25338657002342, -93.35849714429017, -94.3068008800362, -88.27873675614035, -93.30083233782412, -85.39601004639363, -91.46280056925573, -83.25477812069862, -89.43703075785405, -82.62438364466891, -88.2225308674539, -81.04566563419816, -87.59003295267959, -80.9135761936175, -85.77827427186253, -80.22308425470746, -85.54716936739837, -80.30173677397998, -84.2175901500595, -80.56732874040298, -83.37768242883448, -81.48306367425042, -83.8906905917171, -82.20138677185858, -83.36581337182099, -83.25360739403229, -83.86719108117094, -85.13623924398044, -84.60141920705034, -85.63247211425215, -84.61891754501954, -89.11219644534478, -86.93675308563888, -90.65086474060264, -86.91978227755536, -94.32232024107083, -91.1937031528676, -105.67835131078319, -96.01996999749672, -108.19743564556381, -102.1759528334099, -98.13408028328126, -95.42561864673883, -103.03927558417618, -93.13041820570994, -92.61599840933886, -87.41561823576637, -95.6167947640217, -85.45482114157137, -89.26172625327284, -83.64736821155725, -90.73728201983252, -82.95136175993244, -90.47704364999184, -83.00757026802304, -89.1024095672369, -82.29357706840872, -88.23475300940171, -82.03587331514377, -86.85968342180617, -82.35711341553477, -85.81709753106743, -82.79370712523529, -85.95880792378041, -84.08514911178878, -86.24056528669705, -84.26663563351609, -85.11149144200135, -85.48335371583636, -85.92142581813184, -86.91808359752399, -86.58865058087574, -89.98286982647136, -87.49532734785518, -91.95474837719652, -89.34803145467214, -94.49767349488376, -92.45873563416424, -108.8690430269248, -98.69933253742657, -105.06246392868492, -111.38768449697511, -96.99118510161742, -95.28935999072544, -99.57447315645048, -91.921208747929, -94.58067683198153, -89.26115689307557, -95.97632975434266, -87.71112562159823, -95.6026253040889, -86.8643653685995, -94.03413185014664, -84.75458821373303, -90.53152615195356, -84.18265238198386, -90.74003839355723, -83.81237200473785, -88.98630392767043, -83.46732671915824, -88.80833466935512, -84.3729693934194, -89.09540947774846, -84.11269221746572, -87.01477738659764, -85.46574647387061, -88.82633557926184, -85.30529533094341, -86.64432037411572, -88.38882956922036, -89.46178094867575, -88.65167305541695, -89.05173580146197, -90.56355933624823, -89.78350226994066, -93.12832102157176, -91.52067729309718, -99.30869554872353, -94.87507585179671, -103.34143765953752, -100.85184172648087, -122.81434116496578, -106.73815887001018, -100.4378952074342, -102.02001564406744, -97.52306851355098, -94.56940172267517, -96.76524495433301, -89.94805427338399, -97.3848170465787, -88.86035744990033, -94.19234755063327, -86.61835716903454, -91.20282103849767, -85.07595457318845, -91.55874293944323, -85.03788023396316, -91.60457024090475, -84.46215997256039, -90.57121250734171, -84.83435358765959, -90.33972168032196, -84.4873262300197, -89.24140029984238, -85.1352382372926, -88.70896083363503, -85.5975672934432, -89.12875853347873, -86.53505382308096, -89.60175411890748, -88.0071551620068, -89.28181547323886, -89.27126299467224, -89.37796771473032, -91.7125863209184, -91.52209806412742, -93.2645811544421, -91.18984143652762, -95.81363430158875, -93.62301569519619, -104.16775936541315, -104.90602312527591, -113.16700957432688, -116.28917731958283, -101.96572273705183, -98.41482687439297, -99.72098919139918, -94.22144853044513, -95.01564070694563, -94.17707694153272, -94.02287362186925, -89.58355059750363, -98.92261465033643, -89.02859420719695, -94.68073466314038, -86.44103147442705, -91.90373963098203, -86.4749062880022, -94.84153506645869, -86.32943545083764, -91.60215019601517, -86.2323824481995, -92.02155272951049, -85.9972623610034, -91.32387548251664, -85.588514296591, -91.53470648146998, -86.2096134918317, -90.35669055111491, -88.00287392840076, -90.12141751973901, -89.44766457872662, -91.62087976611487, -91.05208067549513, -92.06362797535392, -91.10989004012806, -92.02930632263177, -97.8326419437665, -100.36369914302273, -96.71323750153027, -96.77554535749293, -104.0483458530803, -100.02615902224633, -107.35748572388934, -107.18491846666, -111.2107942940795, -101.34493721885849, -96.18458817889217, -95.05818354852602, -97.34815447051216, -92.36349598065061, -95.78385348959006, -89.7086230203063, -93.2365210743273, -88.04737944359495, -95.39968104514571, -88.1751912031278, -94.33963358398256, -86.96835690829943, -94.3448391909962, -87.94543163312412, -92.90493597746648, -87.22030009538193, -92.61262896853015, -86.30586131244313, -91.96103440057696, -86.7710521640438, -92.10322890271088, -88.8099510544229, -93.31727026496762, -88.39915058817098, -92.9724660735097, -89.53892755878542, -93.5679390287161, -92.14368535308965, -93.89854406383924, -93.06540499762073, -95.3716098006777, -96.36846381712701, -93.63623239819597, -99.39911564797553, -98.40395825782761, -100.94269872968796, -100.48369232950719, -104.96898067375994, -114.335263021867, -101.40187975001979, -98.65627818089435, -106.58072970493392, -104.44376560744413, -95.83027356701794, -92.97753215916143, -101.26434292825368, -93.50367975283709, -93.37263244117777, -89.44861935863923, -95.343734550422, -89.99933130658839, -99.99527004643943, -88.94925644025324, -93.18301244517464, -88.50885338097075, -95.18084024984185, -87.20676030200416, -95.23926810467589, -87.09957224800853, -92.1757639701081, -88.10417272814877, -94.72106133839601, -87.7772108681502, -92.91109610741583, -89.72414668122461, -93.22742894203847, -91.63186037346222, -95.68890880122552, -90.18179583705027, -93.59223328781121, -92.50281370390375, -94.04741609159348, -95.5573835037378, -97.19098591462304, -99.76079766259453, -98.20546781981285, -120.67183723001071, -103.20327161610481, -117.22027024101293, -105.09645279442447, -111.76755429121258, -113.04120386427974, -100.65061200309104, -96.88654432109547, -94.60215846035042, -93.49825828753863, -97.1667542174504, -94.38236741729683, -96.783281591943, -92.939285616442, -95.42524341021134, -89.7310231461323, -96.61418552254929, -89.15181635406329, -93.97977001970317, -89.25630669378194, -99.16812248160959, -89.40549989469969, -97.02103373489075, -88.08117642000238, -96.17212999699518, -87.76166390724612, -93.64057438170258, -88.20421502757773, -94.63414445257587, -89.48275213078753, -92.03704873153879, -91.18822814375747, -94.02753580779823, -92.25046023804195, -94.18472031424919, -95.7912337432503, -97.17361952054567, -97.57189526176677, -96.93431865585318, -102.04551967744064, -98.01984334480733, -97.80936648544454, -96.58319851428925, -103.08073994551233, -110.00167882027728, -108.52196994994446, -105.04853402419212, -101.33233085003278, -100.05040433917165, -99.22073393358865, -97.90929268980324, -98.89113225851989, -94.89288879112064, -97.93384172752636, -93.22419277669928, -96.01960899562502, -90.96253017735826, -94.32065948649546, -90.18255956439114, -94.9243761616897, -88.73145096365911, -95.65826240076106, -90.10091760259287, -98.3156872459785, -88.97172432282879, -94.68357816611993, -89.22286435681411, -96.33113850492892, -90.27256468692858, -97.52356475116345, -92.28994918400562, -96.39548763580854, -90.89270553951194, -95.24683746449244, -92.28348737753878, -94.54135448918169, -92.42301671907596, -96.24508547590521, -99.44340135136264, -100.90085793594595, -101.8210082553093, -100.62139348876947, -107.75005082456524, -101.18792193308998, -100.62321402005587, -106.14445292006377, -105.83949578053429, -107.80632506741767, -102.54660223569036, -108.59151037419879, -96.90782677416453, -100.64769899514724, -98.90076837905437, -96.2725953153946, -100.63869480989204, -93.57497128631536, -97.48996544980523, -92.0598771078806, -97.43531529596639, -91.70896750245781, -97.62553199959177, -89.90453042801695, -98.1895558530371, -91.28563260418011, -96.58606769664732, -89.6602652167721, -97.63127451658008, -90.06188532337133, -96.88320254636814, -92.10434711550748, -102.83415328605342, -91.97522523546786, -96.69674529333655, -91.54555505247494, -96.45677376279522, -94.40105972915326, -99.06442453405175, -95.85784268220618, -100.11209838032768, -96.3666970525114, -100.25033668665256, -101.63701920876531, -101.33176509769909, -108.49220907293285, -105.20698869391131, -108.51201611499555, -110.56213658974848, -103.88286882354619, -107.29652775251672, -100.21199149373265, -102.84474849090422, -105.38837926677445, -101.63659463064025, -100.19927788160382, -95.8841790949619, -99.06159894948496, -93.83003777289345, -98.62241277299339, -93.41972484372512, -96.85163908187218, -92.22305012467251, -98.30931966050954, -91.01393465151821, -96.6610842279197, -93.01366348474153, -99.40254068724771, -91.98688250178945, -97.8197024210045, -90.34022028730962, -95.26212499971268, -90.48623787418245, -97.28501156955554, -93.02707841894987, -99.4242294058617, -93.78403579509337, -102.4058010943352, -92.81743718612427, -97.25554725609649, -97.04610938164143, -104.56111849036819, -101.9867276361093, -103.69614871490393, -104.74168040294428, -100.60066394657342, -102.48071416087461, -104.83064451058839, -107.26658041556234, -110.00503214084297, -103.90297408190925, -109.56149727793942, -103.52026679181287, -103.90051784161805, -102.01215965881818, -103.34803834159351, -98.0276145235799, -96.38035775134539, -97.3546077254475, -94.31453760099365, -99.30006326184404, -96.25250684947787, -96.12470450005495, -91.57830601960927, -94.56483812993685, -91.7611403679199, -100.05865004766831, -92.84402279338929, -95.8657101518119, -91.81837191684286, -96.8413097745885, -89.99396126510099, -100.6611154167793, -93.47882774662997, -101.6552886734432, -91.90487651880966, -97.29970250454008, -95.48622404677303, -100.41640918017757, -94.80515000968441, -98.5276945872201, -100.73609481029864, -98.04340547902302, -96.88540783402982, -103.44300868430581, -99.6601137575993, -104.35594220885358, -109.94922945338091, -109.10632479160674, -107.76641232941655, -105.2450226453189, -99.91265402083279, -99.95270124336952, -101.3299547913052, -99.96894232524801, -100.36365349460627, -102.86784602376038, -98.02737777122191, -96.17199616892495, -96.8931790371181, -95.96337763969792, -97.57196266275315, -95.0155693239098, -97.04855005360989, -94.47249259707691, -99.4517730137364, -92.94791202171595, -97.78312777875891, -94.30168526906485, -94.86398262799752, -93.54115309153002, -99.87583067187317, -92.51726891229963, -102.13604597983688, -92.17994531242135, -101.63856277413217, -95.35318079876619, -99.29709984960036, -95.35866979801156, -103.51166947626271, -94.86370220831154, -101.60407867882681, -103.74156718150365, -110.73370380070999, -103.71760139847281, -107.37490721838113, -109.9542240510403, -116.25403765775846, -108.23241740959084, -105.09846687198814, -105.44052253244195, -115.24118791748435, -103.49001515992114, -110.71286352533042, -105.89441442611357, -110.16493279526881, -99.82773652058825, -98.97179081977004, -98.45757481371732, -98.24962705928117, -96.73193799282699, -96.5175230963137, -96.15492740611579, -95.37412981355675, -103.58492432555138, -95.34117451236305, -97.11997617370957, -93.47520800696678, -110.25299719363927, -96.81885358127444, -99.9145312135518, -94.20482495341496, -98.89579295580432, -93.36303704542247, -100.68935843408086, -93.24714444319031, -100.69789100599222, -95.91175346020901, -104.76997205430096, -94.51143912041329, -100.54159089868858, -102.05805669840157, -99.78073889500477, -95.8994839656266, -104.44581361115654, -97.35459561709312, -102.43458217795424, -99.94756951585332, -116.63154202021275, -104.67083143207799, -105.9908001506922, -110.38171109041919, -112.65697869449573, -108.99847694028415, -108.57898585331196, -104.24393364688189, -105.73441833654073, -109.05313569411014, -109.36295935913135, -98.16710161937883, -100.71703118273305, -99.09017072666417, -99.65556811710037, -99.82196229518456, -96.7135911059506, -102.93949494534098, -98.73450476723507, -97.07204978552434, -94.0346238995044, -101.15510126297552, -96.31490423262902, -97.71794077324151, -95.06125394279763, -97.42135900154832, -93.74600546845856, -114.1734093772797, -94.81930930716295, -97.06186795913504, -97.8835566026099, -103.92592509446062, -93.22500956494437, -99.20608880696017, -96.85801972443574, -107.87319613965472, -95.4606711561285, -109.77479647459404, -101.94651160973874, -109.21384119060488, -103.26877357606884, -104.34360525896628, -103.21689879150107, -103.51193808052379, -110.73067516385558, -106.23572152985658, -100.40039512525607, -104.4691097545222, -101.492896976522, -108.0496930826297, -104.38836363424356, -103.20083256140792, -98.90311658646465, -112.5916141563029, -97.44686284058668, -98.65253112982872, -97.56094346469311, -99.80658861772346, -99.20048346610903, -96.35632860142131, -99.28522795713639, -98.60285966904206, -97.78263171380898, -95.6007337511918, -103.2099329489675, -95.38702929874557, -102.13771129182885, -95.14930315850044, -98.3128670125364, -92.63546383992049, -104.71027133304193, -96.912283335093, -108.90993472372125, -99.55733899189684, -105.52550816632844, -97.40882660368159, -104.42281900752256, -99.57292672864625, -100.7966736295322, -97.52156624066522, -99.99073018359479, -99.0509840665854, -101.68754399107273, -101.12194458233189, -102.0463932610904, -105.91609044634541, -113.23554586573385, -101.98602750398949, -105.2635176386883, -103.79769775471262, -105.9111241296442, -107.9342434738976, -100.92121390473184, -97.12092290766883, -102.37764998835347, -98.6487783972021, -106.87222299917964, -99.33800557071586, -101.79953571256968, -100.91730518889514, -98.78879349468048, -98.23175546624212, -97.00117266559471, -101.37082956877207, -96.83259964822547, -104.87830362769942, -98.16713025626292, -101.96039957310882, -96.50507041796234, -101.8071196906989, -95.79349732553376, -102.02735914214256, -97.56201616761655, -103.1907064807159, -100.09953975957055, -112.56599817646672, -96.53563750179535, -99.9094561567417, -104.40141402751925, -115.46650328556561, -99.71467979897997, -102.79169020107405, -115.69624536220817, -100.76234254160234, -101.71038578591319, -103.75525178434926, -109.55422465835552, -106.65763594732093, -100.05230601631467, -102.10477478530564, -107.51891686962597, -114.58223661159585, -103.67146489337358, -101.5653675539541, -102.32103991938665, -103.67558252237892, -105.48352665247177, -109.55108760057558, -100.02982943314349, -98.13628340653156, -99.47346703290722, -98.92228326973435, -106.95782992135295, -105.89070869451947, -100.44660814326556, -97.09766369078704, -107.64297990254909, -105.84369355013555, -99.08393974061082, -96.374032771269, -102.65269590892945, -97.64870380479474, -105.90868162170571, -96.9898469284162, -105.2441700741264, -106.53146741239493, -106.46615178101108, -99.37447573772154, -109.39976410894721, -104.62921354447154, -101.87865689170566, -101.32860591590756, -114.43680707235822, -106.46190634887617, -113.36934474874106, -112.67163951557576, -102.66437005552562, -101.59964732308622, -122.77511747329424, -105.70845427584239, -108.46107323638913, -122.08650568486307, -111.16233468390396, -105.6496162612092, -105.79716011047833, -109.29698973600742, -106.5972312190114, -106.38945639217272, -105.63454774600953, -110.2830820244838, -105.77280978659724, -108.93057545365407, -109.17523925675454, -104.7131107168997, -103.60696199900858, -102.73166871321888, -97.49220135377621, -99.78808799700637, -101.11339791104449, -105.3939613260955, -103.42765288248593, -105.9340205661671, -107.77841485489014, -112.54860851403683, -120.22611245470668, -103.24971407964512, -104.3429544521227, -107.19732309503469, -107.16251497679025, -108.44664442280767, -101.62190077250342, -111.55917555022586, -104.81037871139557, -102.19463977156316, -105.04595625851906, -111.13196253104579, -124.72753891569215, -106.41597417621414, -105.12116350513813, -109.07754889691405, -105.23915229069101, -100.2688134501812, -107.02689810915471, -109.80290323096122, -103.81257666065085, -103.93774311881742, -110.756399743658, -111.62163187481585, -104.70396973658701, -110.06008823269457, -102.37808137382835, -103.60682103116714, -108.7695179644936, -102.98806816979182, -108.95209477982092, -102.75152787003978, -110.5775345178838, -107.60670935161642, -111.40615158129323, -109.13401107224777, -116.61575163192845, -107.96409706790726, -107.25727436770623, -101.17937824997462, -101.48759426936303, -101.66993276693202, -108.51517738724363, -111.89027836420303, -105.82817808958634, -106.26049115128238, -115.0445929460676, -109.17008677215136, -110.56032445093282, -113.06962595211048, -104.72451144495747, -103.61986219276268, -103.93451254257806, -131.06358095275755, -105.10487085176783, -105.25246852224541, -106.12903690082682, -107.23522918531137, -106.27438688637619, -107.07518949090365, -106.0552389825976, -103.69306509532366, -103.41067687310449, -105.62796514613967, -105.09396645540701, -104.41575397097671, -106.21837017613421, -109.37322036445215, -107.2496046853047, -121.3348235662606, -111.11906633319107, -111.8877022511887, -112.63080142659376, -108.83825637747428, -106.2095359458504, -119.63268129656143, -123.9219371113987, -111.93522459359046, -111.31094152610274, -105.26691970177436, -106.04931130074439, -116.50378960248553, -113.82805948415167, -114.82071561851546, -107.43149967133049, -103.03687243275733, -101.63522623347686, -102.80934641992253, -107.82093212276692, -114.84037503828779, -112.35787341855624, -109.53816987092426, -102.9999489914469, -107.89601039792339, -106.37583865949857, -109.67283710223154]}, ...(4 in all)]
  in  "app.quit":bool
  in  "lock-in.boxcar length 0":u32=2048 caption="Boxar Length"
  in  "app.tab 0":enum32{"Lock-In", "PLL", "Output"}(tab)
  in  "lock-in.manual carrier 0":dbl=100000.0 caption="Carrier" format="%#_6p"
  in  "lock-in.decimation 0":i32=8192 caption="Decimation" min=8 max=8192
  in  "lock-in.source 0":enum16{"AI 0", "AI 1", "AI 2", "AI 3"}(ring)=enum."AI 1" caption="Channel"
  in  "lock-in.carrier 0":T2(ring)=enum."PLL 0" caption="Carrier Source"
  in  "pll.m 0":i8=-27 caption="M"
  in  "pll.source 0":enum16{"AI 0", "AI 1", "AI 2", "AI 3"}(ring) caption="Source"
  in  "pll.q frequency 0":dbl=100000.0 caption="Q Frequency" format="%#_6p"
  in  "pll.reset 0":bool
  in  "ao.noise 3":dbl caption="A0 3 Noise" min=0.0 max=1.0 format="%#_6p"
  in  "ao.level 3":dbl=0.5 caption="A0 3 Level" format="%#_6pV"
  in  "ao.frequency 3":dbl=10000000.0 caption="AO 3 Frequency" format="%#.9p"
  in  "ao.frequency 0":dbl=10000000.0 caption="AO 0 Frequency" format="%#.9p"
  in  "ao.level 0":dbl=0.5 caption="AO 0 Level" format="%#_6pV"
  in  "rio device":tag="PXI1Slot4" caption="Resource"
  in  "lock-in.reset boxar 0":bool
  out "lock-in.deviation 1":dbl caption="Deviation" format="%#_6p"
  out "lock-in.amplitude 0":dbl caption="Result" format="%#_6p"
  in  "lock-in.boxcar lookback 0":i32=1024 caption="Windows to Average"
  out "Result":cluster{"mean":dbl, "trace":dbl}(graph)
  # "NI Lock-In Amplifier Reference Example"
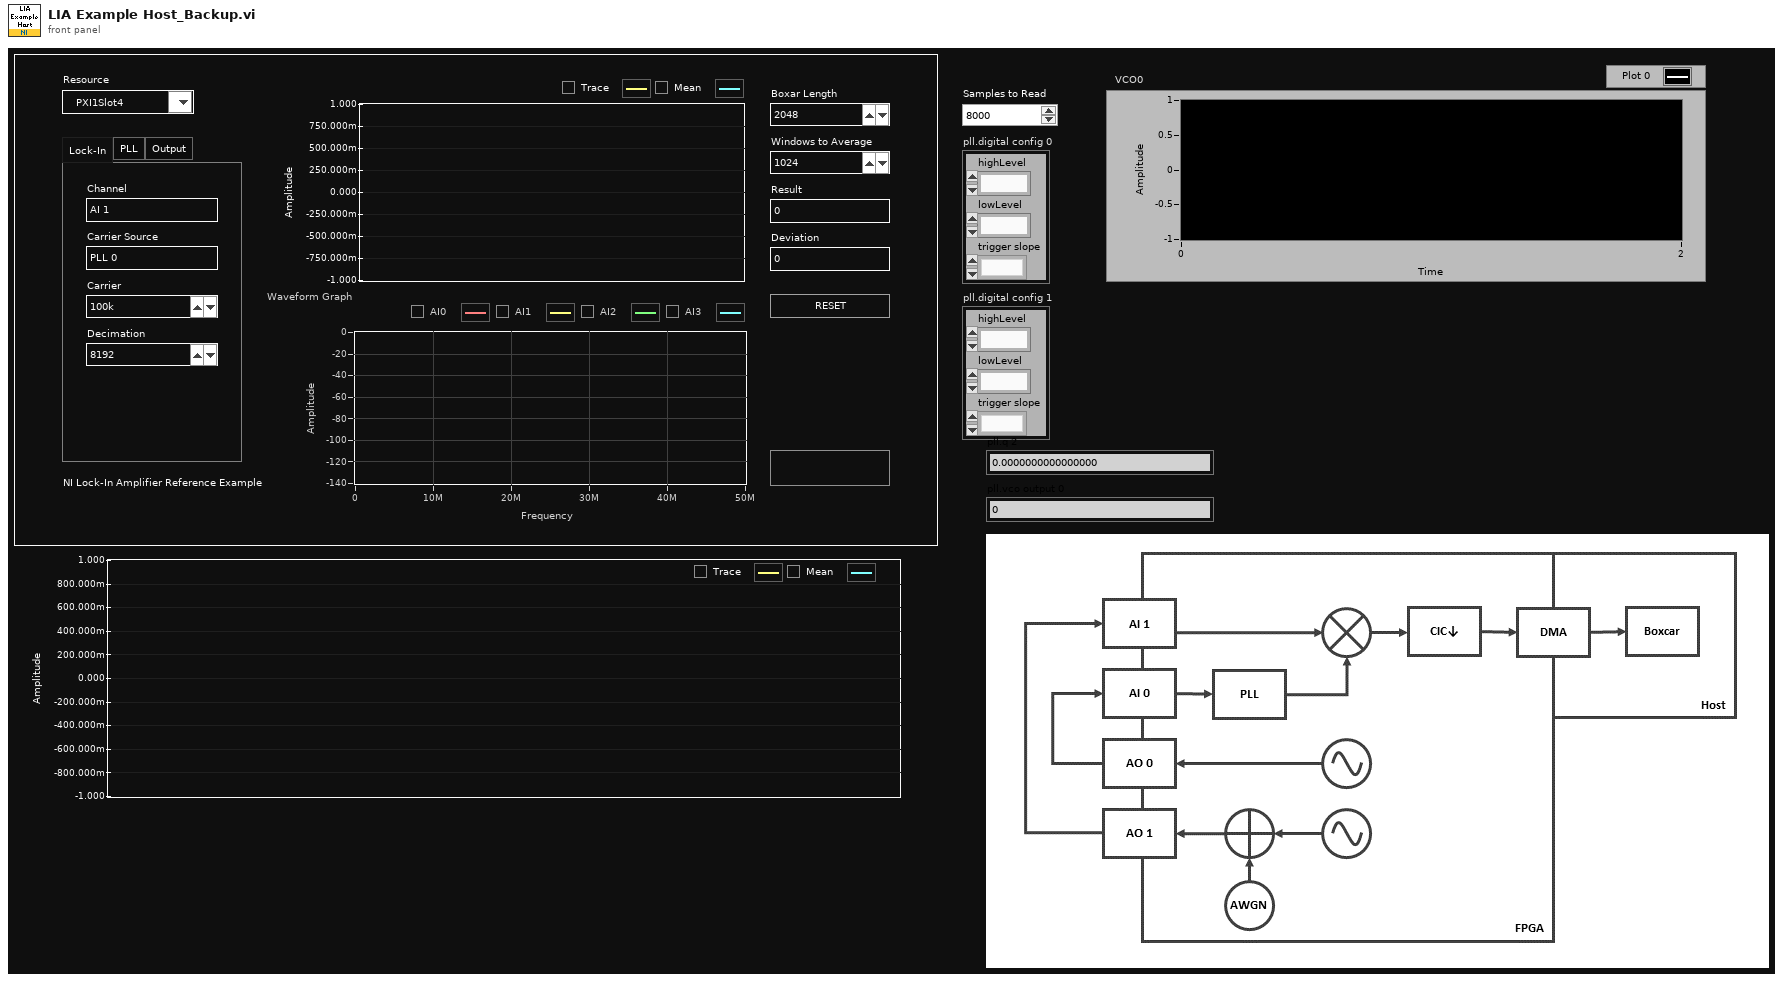
[diagram p1: front panel]
types:
  T1 = cluster{"highLevel":fxp<+/-,18,1>, "lowLevel":fxp<+/-,18,1>, "trigger slope":enum8{"Positive", "Negative"}}
  T2 = enum16{"Manual 0", "Manual 1", "Manual 2", "Manual 3", "PLL 0", "PLL 1"}
  T3 = typedef "Lock-In Amplifier Example Host.lvlib/lock-in settings.ctl" = cluster{"decimation":i32, "source":i32, "carrier source":i32, "carrier":dbl}
  T4 = typedef "Lock-In Amplifier Example Host.lvlib/pll settings.ctl" = cluster{"source":i32, "q frequency":dbl}
  T5 = typedef "Lock-In Amplifier Example Host.lvlib/fpga type.ctl" = refnum<k20>
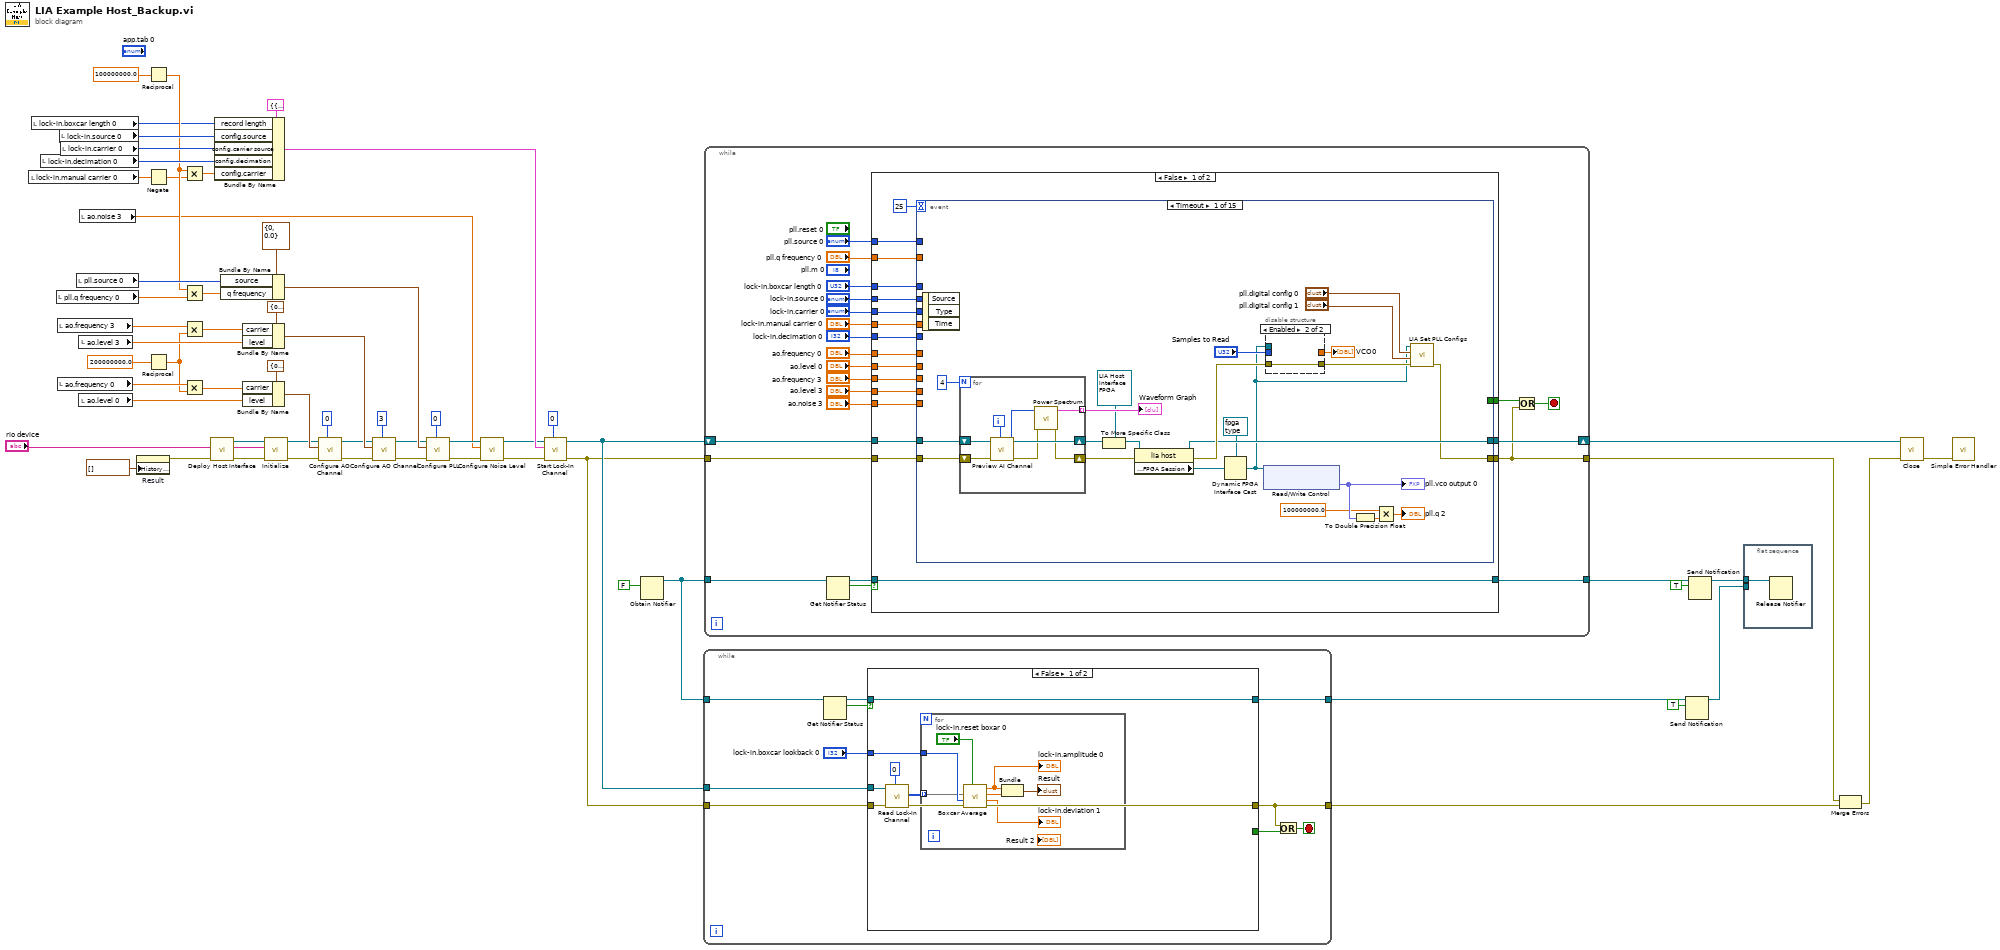
[diagram p0: block diagram]
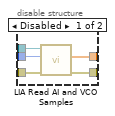
[diagram p2: hidden frame]
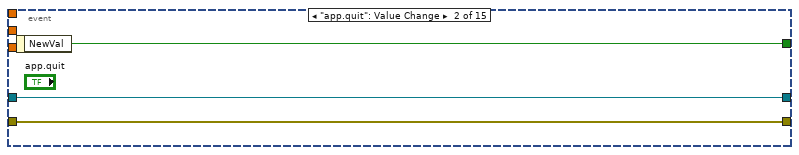
[diagram p3: hidden frame]
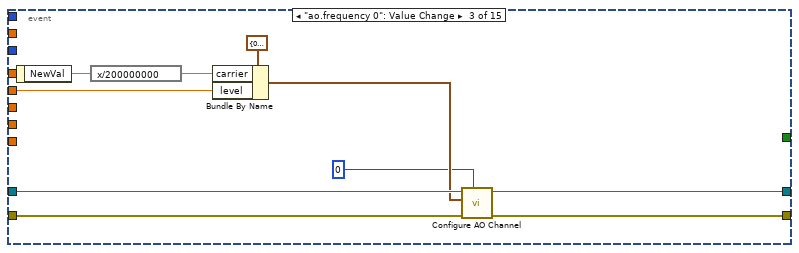
[diagram p4: hidden frame]
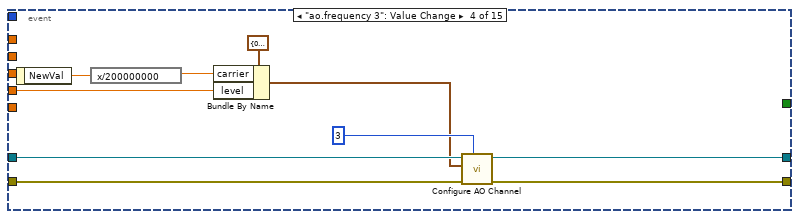
[diagram p5: hidden frame]
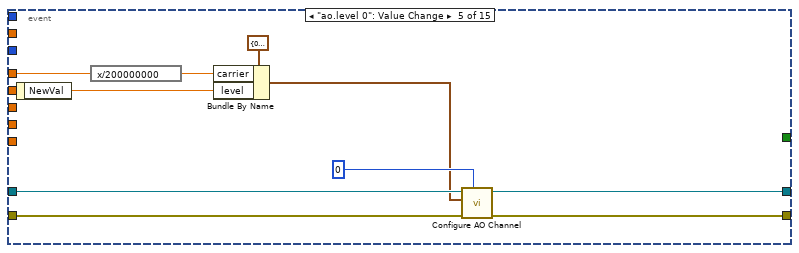
[diagram p6: hidden frame]
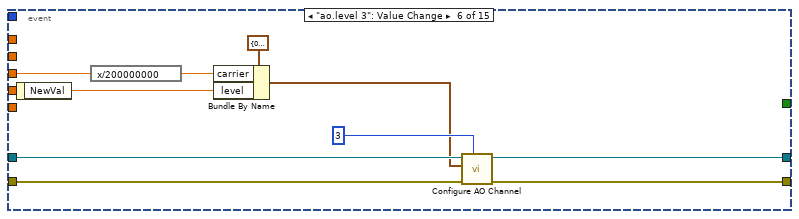
[diagram p7: hidden frame]
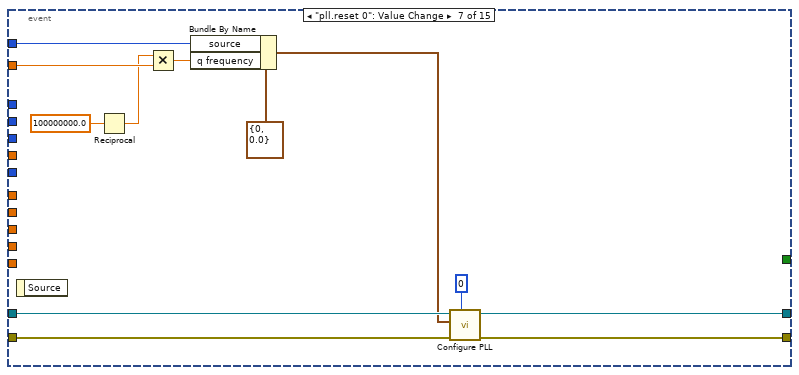
[diagram p8: hidden frame]
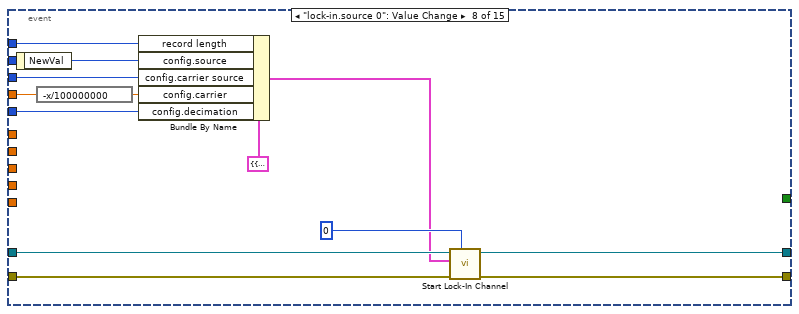
[diagram p9: hidden frame]
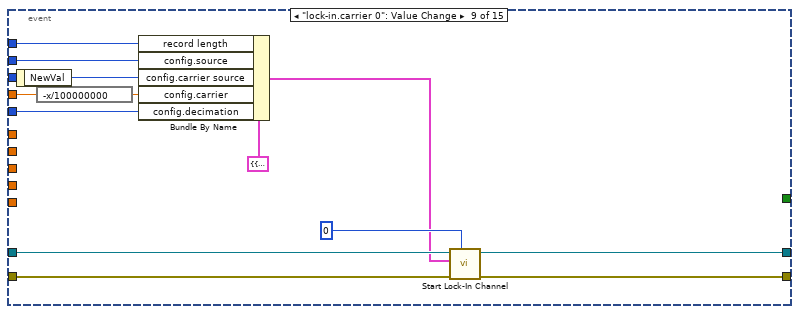
[diagram p10: hidden frame]
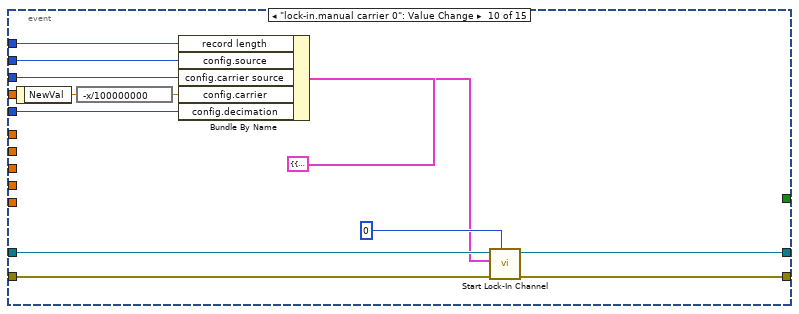
[diagram p11: hidden frame]
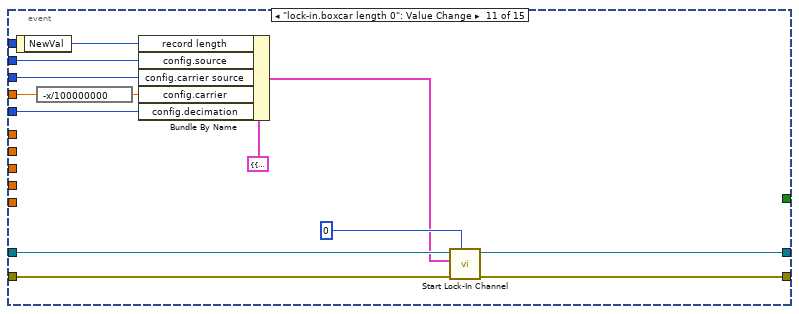
[diagram p12: hidden frame]
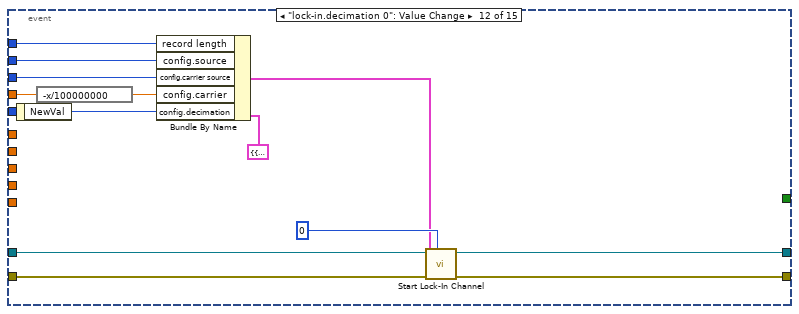
[diagram p13: hidden frame]
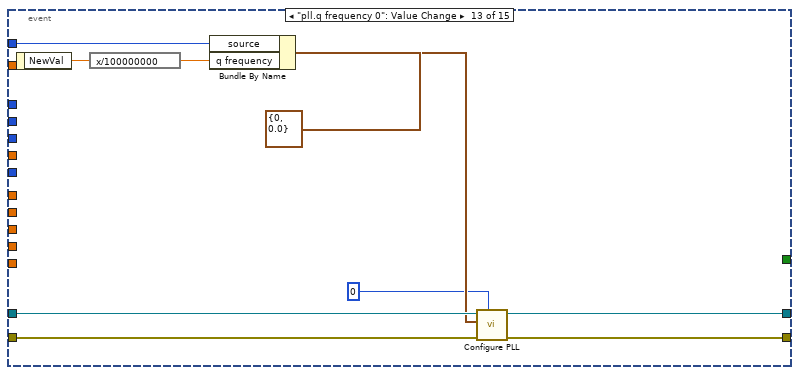
[diagram p14: hidden frame]
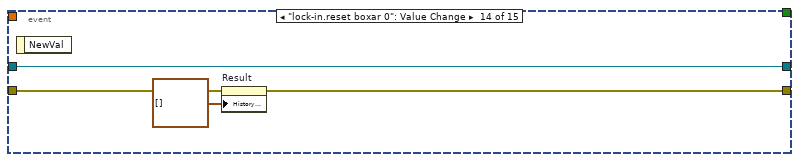
[diagram p15: hidden frame]
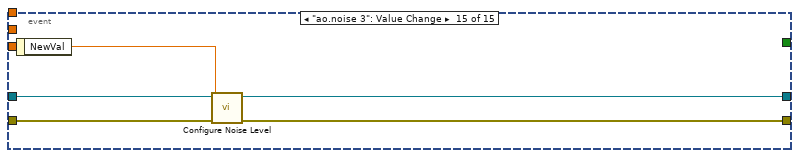
[diagram p16: hidden frame]
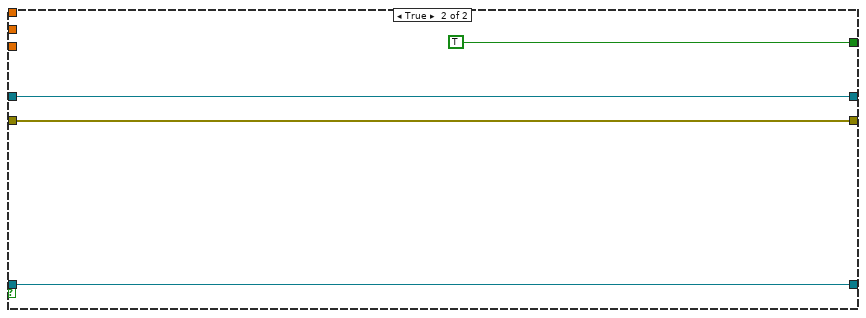
[diagram p17: hidden frame]
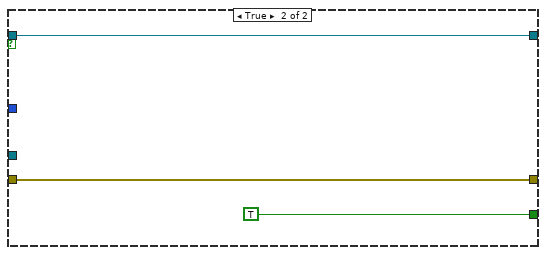
[diagram p18: hidden frame]
diagram:
  n1 = local read "lock-in.manual carrier 0"() -> (w50:dbl)
  n2 = local read "lock-in.boxcar length 0"() -> (w14:u32)
  n3 = local read "lock-in.decimation 0"() -> (w53:i32)
  n4 = local read "pll.q frequency 0"() -> (w55:dbl)
  n5 = local read "ao.frequency 3"() -> (w47:dbl)
  n6 = local read "ao.frequency 0"() -> (w44:dbl)
  n7 = local read "lock-in.source 0"() -> (w64:enum16{"AI 0", "AI 1", "AI 2", "AI 3"})
  n8 = local read "lock-in.carrier 0"() -> (w63:T2)
  n9 = local read "pll.source 0"() -> (w61:enum16{"AI 0", "AI 1", "AI 2", "AI 3"})
  n10 = local read "ao.level 3"() -> (w59:dbl)
  n11 = local read "ao.level 0"() -> (w58:dbl)
  n12 = local read "ao.noise 3"() -> (w3:dbl)
  n13 = property on="Result" class="WFChart (strict)"("History Data"=cluster{"mean":dbl, "trace":dbl}[] []) -> (error out=w9:errorcluster)  [unwired: 2 in, 1 out]
  n14 = Reciprocal(x=100000000.0) -> (1/x=w51:dbl)
  n15 = Negate(x=w50) -> (-x=w49:dbl)
  n16 = Reciprocal(x=200000000.0) -> (1/x=w43:dbl)
  n17 = Multiply(x=w51, y=w49) -> (x*y=w52:dbl)
  n18 = Multiply(x=w51, y=w55) -> (x*y=w56:dbl)
  n19 = Multiply(x=w47, y=w43) -> (x*y=w48:dbl)
  n20 = Multiply(x=w44, y=w43) -> (x*y=w45:dbl)
  n21 = call "Deploy Host Interface.vi"("error in"=w9, "resource"="rio device") -> ("error out"=w10:errorcluster, "resource out"=w11:string, "lia host interface"=w12:refnum<class "LIA Host Interface.lvclass">)  [unwired: 7 in]
  n22 = Bundle By Name(cluster=cluster{"config":T3, "record length":u32} {"config"={"decimation"=0, "source"=0, "carrier source"=0, "carrier"=0.0}, "record length"=0} ("config"), "record length"=w14, "config.source"=w64, "config.carrier source"=w63, "config.decimation"=w53, "config.carrier"=w52) -> (w15:cluster{"config":T3, "record length":u32})
  n23 = Bundle By Name(cluster=T4 {"source"=0, "q frequency"=0.0} ("config"), "source"=w61, "q frequency"=w56) -> (w40:T4)
  n24 = Bundle By Name(cluster=cluster{"carrier":dbl, "level":dbl} {"carrier"=0.0, "level"=0.0} ("config"), "carrier"=w48, "level"=w59) -> (w41:cluster{"carrier":dbl, "level":dbl})
  n25 = Bundle By Name(cluster=cluster{"carrier":dbl, "level":dbl} {"carrier"=0.0, "level"=0.0} ("config"), "carrier"=w45, "level"=w58) -> (w42:cluster{"carrier":dbl, "level":dbl})
  n26 = call-dynamic "Initialize.vi"("error in"=w10, "resource"=w11, "lia host in"=w12) -> ("error out"=w24:errorcluster, "lia host out"=w25:refnum<class "LIA Host Interface.lvclass">)  [unwired: 7 in]
  n27 = call-dynamic "Configure AO Channel.vi"("instance"=0 ("index"), "error in"=w24, "config"=w42, "lia host in"=w25) -> ("error out"=w23:errorcluster, "lia host out"=w22:refnum<class "LIA Host Interface.lvclass">)  [unwired: 6 in]
  n28 = call-dynamic "Configure AO Channel.vi"("instance"=3 ("index"), "error in"=w23, "config"=w41, "lia host in"=w22) -> ("error out"=w18:errorcluster, "lia host out"=w19:refnum<class "LIA Host Interface.lvclass">)  [unwired: 6 in]
  n29 = call-dynamic "Configure PLL.vi"("instance"=0 ("index"), "error in"=w18, "config"=w40, "lia host in"=w19) -> ("error out"=w7:errorcluster, "lia host out"=w4:refnum<class "LIA Host Interface.lvclass">)  [unwired: 6 in]
  n30 = call-dynamic "Configure Noise Level.vi"("error in"=w7, "level"=w3, "lia host in"=w4) -> ("error out"=w6:errorcluster, "lia host out"=w5:refnum<class "LIA Host Interface.lvclass">)  [unwired: 7 in]
  n31 = call-dynamic "Start Lock-In Channel.vi"("instance"=0 ("index"), "error in"=w6, "config"=w15, "lia host in"=w5) -> ("error out"=w35:errorcluster, "lia host out"=w36:refnum<class "LIA Host Interface.lvclass">)  [unwired: 6 in]
  n32 = Obtain Notifier(notification data type=FALSE) -> (notifier out=w37:refnum<notifier>)  [unwired: 3 in, 2 out]
  n33 = while {
    tunnel: w37 -> [w74]
    tunnel: w36 -> [w71]
    tunnel: w35 -> [w70]
    tunnel: [w69] -> w28
    tunnel: [w66] -> w31
    stop <- w68 stop-if-true
    n34 = Get Notifier Status(notifier=w74) -> (notifier out=w72:refnum<notifier>, current notification=w73:bool)  [unwired: 1 in, 3 out]
    n35 = case shown="False" w73 {
      tunnel: [w78 w91] -> w66
      tunnel: w72 -> [w78 w91]
      tunnel: w71 -> [w81 _]
      tunnel: w70 -> [w80 w90]
      tunnel: [w77 w90] -> w69
      tunnel: [_ TRUE] -> w67
      tunnel: "lock-in.boxcar lookback 0" -> [w76 _]
      frame False {
        n36 = call-dynamic "Read Lock-In Channel.vi"("instance"=0 ("index"), "error in"=w80, "lia host in"=w81) -> ("error out"=w77:errorcluster, "unscaled data"=w75:i64[][])  [unwired: 6 in, 1 out]
        n37 = for {
          tunnel: w75 -> [w83] mode=indexing
          tunnel: w76 -> [w84]
          n38 = call "Boxcar Average.vi"("reset"="lock-in.reset boxar 0", "sample length"=w84, "interleaved iq"=w83) -> ("standard deviation"=→"lock-in.deviation 1":dbl, "trace"=w88:dbl, "mean"=w85:dbl)  [unwired: 6 in]
          "lock-in.amplitude 0" <- w85
          n39 = Bundle("mean"=w85, "trace"=w88) -> (→"Result":cluster{"mean":dbl, "trace":dbl})  [unwired: 1 in]
        }
      }
      frame True {
      }
    }
    n40 = Or(x=w69, y=w67) -> (x .or. y?=w68:bool)
  }
  n41 = while {
    tunnel: w35 -> [w113]
    shift-right: [w99] -> w39
    shift-left: w36 -> [w112]
    tunnel: [w95] -> w27
    tunnel: w37 -> [w98]
    tunnel: [w93] -> w34
    stop <- w111 stop-if-true
    n42 = Get Notifier Status(notifier=w98) -> (notifier out=w97:refnum<notifier>, current notification=w96:bool)  [unwired: 1 in, 3 out]
    n43 = case shown="False" w96 {
      tunnel: w113 -> [w132 w311]
      tunnel: w112 -> [w131 w312]
      tunnel: [w130 w311] -> w95
      tunnel: "lock-in.manual carrier 0" -> [w128 _]
      tunnel: "lock-in.decimation 0" -> [w127 _]
      tunnel: "lock-in.source 0" -> [w126 _]
      tunnel: "lock-in.carrier 0" -> [w125 _]
      tunnel: "pll.source 0" -> [w124 _]
      tunnel: "pll.q frequency 0" -> [w123 _]
      tunnel: "ao.frequency 0" -> [w122 _]
      tunnel: "ao.level 0" -> [w121 _]
      tunnel: "ao.frequency 3" -> [w120 _]
      tunnel: "ao.level 3" -> [w119 _]
      tunnel: "ao.noise 3" -> [w118 _]
      tunnel: [w117 w312] -> w99
      tunnel: w97 -> [w115 w309]
      tunnel: [w116 TRUE] -> w94
      tunnel: [w115 w309] -> w93
      tunnel: "lock-in.boxcar length 0" -> [w114 _]
      frame False {
        n44 = event shown="[0] Timeout" {
          selector: _ -> [_ _ _ _ _ _ _ _ _ _ _ _ _ _ _]
          dyn-events: _ -> [_ _ _ _ _ _ _ _ _ _ _ _ _ _ _]
          timeout: 25 -> [_ _ _ _ _ _ _ _ _ _ _ _ _ _ _]
          tunnel: w132 -> [w153 w171 w177 w192 w202 w212 w224 w233 w247 w260 w272 w286 w295 w303 w307]
          tunnel: w131 -> [w154 w172 w178 w191 w201 w211 w223 w231 w245 w258 w270 w284 w294 w300 w308]
          tunnel: [w141 w171 w175 w190 w200 w210 w222 w232 w246 w259 w271 w285 w292 w302 w305] -> w130
          tunnel: w126 -> [_ _ _ _ _ _ _ _ w238 w251 w264 w280 _ _ _]
          tunnel: w125 -> [_ _ _ _ _ _ _ w236 _ w262 w275 w288 _ _ _]
          tunnel: w128 -> [_ _ _ _ _ _ _ w235 w249 _ w274 w287 _ _ _]
          tunnel: w127 -> [_ _ _ _ _ _ _ w234 w248 w261 w273 _ _ _ _]
          tunnel: w124 -> [_ _ _ _ _ _ w217 _ _ _ _ _ w297 _ _]
          tunnel: w123 -> [_ _ _ _ _ _ w218 _ _ _ _ _ _ _ _]
          tunnel: w122 -> [_ _ _ _ w195 _ _ _ _ _ _ _ _ _ _]
          tunnel: w121 -> [_ _ w180 _ _ _ _ _ _ _ _ _ _ _ _]
          tunnel: w120 -> [_ _ _ _ _ w205 _ _ _ _ _ _ _ _ _]
          tunnel: w119 -> [_ _ _ w185 _ _ _ _ _ _ _ _ _ _ _]
          tunnel: w118 -> [_ _ _ _ _ _ _ _ _ _ _ _ _ _ _]
          tunnel: [w148 w172 w173 w183 w193 w203 w213 w230 w244 w257 w269 w283 w293 w300 w306] -> w117
          tunnel: [_ w170 _ _ _ _ _ _ _ _ _ _ _ _ _] -> w116
          tunnel: w114 -> [_ _ _ _ _ _ _ w226 w241 w254 _ w278 _ _ _]
          event Timeout {
            n45 = event-data() -> ()  [unwired: 1 in, 3 out]
            n46 = for {
              N: 4 -> [_]
              shift-right: [w167] -> w149
              shift-left: w154 -> [w169]
              shift-right: [w164] -> w152
              shift-left: w153 -> [w168]
              tunnel: [w162] -> w150 mode=indexing
              i -> [w166]
              n47 = call-dynamic "Preview AI Channel.vi"("instance"=w166, "error in"=w168, "lia host in"=w169) -> ("error out"=w165:errorcluster, "samples"=w163:i16[], "lia host out"=w167:refnum<class "LIA Host Interface.lvclass">)  [unwired: 6 in]
              n48 = call "Power Spectrum.vi"("error in"=w165, "ai data"=w163) -> ("error out"=w164:errorcluster, "magnitude"=w162:cluster{"f0":dbl, "df":dbl, "magnitude":dbl[]})  [unwired: 8 in]
            }
            "Waveform Graph" <- w150
            n49 = To More Specific Class(target class=refnum<class "LIA Host Interface FPGA.lvclass"> refnum ("lia host"), reference=w149) -> (specific class reference=w147:refnum<class "LIA Host Interface FPGA.lvclass">)  [unwired: 1 in, 1 out]
            n50 = property class="lia host"(reference=w147, error in=w152) -> (reference out=w148:refnum<class "LIA Host Interface FPGA.lvclass">, error out=w155:errorcluster, "Properties:FPGA Session"=w145:refnum<k20>)
            n51 = Dynamic FPGA Interface Cast(Session In=T5 refnum ("fpga type"), Type=w145) -> (Session Out=w138:T5)
            n52 = xnode "Read/Write Control"("FPGA VI Reference In"=w138) -> ("pll.vco output 0"=w135:fxp<+/-,49,1>)  [unwired: 1 in, 2 out]
            "pll.vco output 0" <- w135
            n53 = disable-structure shown="Enabled" {
              disable-tunnel: w155 -> [w160 w161]
              disable-tunnel: "Samples to Read" -> [w159 _]
              disable-tunnel: [w158 w161] -> w142
              disable-tunnel: w138 -> [w157 _]
              disable-tunnel: [w156 _] -> w133
              frame Disabled {
                n54 = call "LIA Read AI and VCO Samples.vi"("error in (no error)"=w160, "samples to read"=w159, "fpga session in"=w157) -> ("error out"=w158:errorcluster, "VCO"=w156:dbl[])  [unwired: 6 in, 1 out]
              }
              frame Enabled {
              }
            }
            "VCO0" <- w133
            n55 = To Double Precision Float(number=w135) -> (double precision float=w136:dbl)
            n56 = Multiply(x=100000000.0, y=w136) -> (x*y=→"pll.q 2":dbl)
            n57 = call "LIA Set PLL Configs.vi"("error in (no error)"=w142, "pll.digital config 1"="pll.digital config 1", "pll.digital config 0"="pll.digital config 0", "fpga session in"=w138) -> ("error out"=w141:errorcluster)  [unwired: 7 in]
          }
          event "app.quit": Value Change {
            n58 = event-data() -> ("NewVal"=w170:bool)  [unwired: 1 in]
          }
          event "ao.frequency 0": Value Change {
            n59 = event-data() -> ("NewVal"=w179:dbl)  [unwired: 1 in]
            n60 = expression code="x/200000000"(w179) -> (w181:dbl)
            n61 = Bundle By Name(cluster=cluster{"carrier":dbl, "level":dbl} {"carrier"=0.0, "level"=0.0} ("config"), "carrier"=w181, "level"=w180) -> (w176:cluster{"carrier":dbl, "level":dbl})
            n62 = call-dynamic "Configure AO Channel.vi"("instance"=0 ("index"), "error in"=w177, "config"=w176, "lia host in"=w178) -> ("error out"=w175:errorcluster, "lia host out"=w173:refnum<class "LIA Host Interface.lvclass">)  [unwired: 6 in]
          }
          event "ao.frequency 3": Value Change {
            n63 = event-data() -> ("NewVal"=w186:dbl)  [unwired: 1 in]
            n64 = expression code="x/200000000"(w186) -> (w188:dbl)
            n65 = Bundle By Name(cluster=cluster{"carrier":dbl, "level":dbl} {"carrier"=0.0, "level"=0.0} ("config"), "carrier"=w188, "level"=w185) -> (w184:cluster{"carrier":dbl, "level":dbl})
            n66 = call-dynamic "Configure AO Channel.vi"("instance"=3 ("index"), "error in"=w192, "config"=w184, "lia host in"=w191) -> ("error out"=w190:errorcluster, "lia host out"=w183:refnum<class "LIA Host Interface.lvclass">)  [unwired: 6 in]
          }
          event "ao.level 0": Value Change {
            n67 = event-data() -> ("NewVal"=w196:dbl)  [unwired: 1 in]
            n68 = expression code="x/200000000"(w195) -> (w198:dbl)
            n69 = Bundle By Name(cluster=cluster{"carrier":dbl, "level":dbl} {"carrier"=0.0, "level"=0.0} ("config"), "carrier"=w198, "level"=w196) -> (w194:cluster{"carrier":dbl, "level":dbl})
            n70 = call-dynamic "Configure AO Channel.vi"("instance"=0 ("index"), "error in"=w202, "config"=w194, "lia host in"=w201) -> ("error out"=w200:errorcluster, "lia host out"=w193:refnum<class "LIA Host Interface.lvclass">)  [unwired: 6 in]
          }
          event "ao.level 3": Value Change {
            n71 = event-data() -> ("NewVal"=w206:dbl)  [unwired: 1 in]
            n72 = expression code="x/200000000"(w205) -> (w208:dbl)
            n73 = Bundle By Name(cluster=cluster{"carrier":dbl, "level":dbl} {"carrier"=0.0, "level"=0.0} ("config"), "carrier"=w208, "level"=w206) -> (w204:cluster{"carrier":dbl, "level":dbl})
            n74 = call-dynamic "Configure AO Channel.vi"("instance"=3 ("index"), "error in"=w212, "config"=w204, "lia host in"=w211) -> ("error out"=w210:errorcluster, "lia host out"=w203:refnum<class "LIA Host Interface.lvclass">)  [unwired: 6 in]
          }
          event "pll.reset 0": Value Change {
            n75 = event-data() -> ()  [unwired: 1 in, 1 out]
            n76 = Reciprocal(x=100000000.0) -> (1/x=w215:dbl)
            n77 = Multiply(x=w215, y=w218) -> (x*y=w220:dbl)
            n78 = Bundle By Name(cluster=T4 {"source"=0, "q frequency"=0.0} ("config"), "source"=w217, "q frequency"=w220) -> (w214:T4)
            n79 = call-dynamic "Configure PLL.vi"("instance"=0 ("index"), "error in"=w224, "config"=w214, "lia host in"=w223) -> ("error out"=w222:errorcluster, "lia host out"=w213:refnum<class "LIA Host Interface.lvclass">)  [unwired: 6 in]
          }
          event "lock-in.source 0": Value Change {
            n80 = event-data() -> ("NewVal"=w228:enum16{"AI 0", "AI 1", "AI 2", "AI 3"})  [unwired: 1 in]
            n81 = expression code="-x/100000000"(w235) -> (w237:dbl)
            n82 = Bundle By Name(cluster=cluster{"config":T3, "record length":u32} {"config"={"decimation"=0, "source"=0, "carrier source"=0, "carrier"=0.0}, "record length"=0} ("config"), "record length"=w226, "config.source"=w228, "config.carrier source"=w236, "config.carrier"=w237, "config.decimation"=w234) -> (w225:cluster{"config":T3, "record length":u32})
            n83 = call-dynamic "Start Lock-In Channel.vi"("instance"=0 ("index"), "error in"=w233, "config"=w225, "lia host in"=w231) -> ("error out"=w232:errorcluster, "lia host out"=w230:refnum<class "LIA Host Interface.lvclass">)  [unwired: 6 in]
          }
          event "lock-in.carrier 0": Value Change {
            n84 = event-data() -> ("NewVal"=w239:T2)  [unwired: 1 in]
            n85 = expression code="-x/100000000"(w249) -> (w250:dbl)
            n86 = Bundle By Name(cluster=cluster{"config":T3, "record length":u32} {"config"={"decimation"=0, "source"=0, "carrier source"=0, "carrier"=0.0}, "record length"=0} ("config"), "record length"=w241, "config.source"=w238, "config.carrier source"=w239, "config.carrier"=w250, "config.decimation"=w248) -> (w240:cluster{"config":T3, "record length":u32})
            n87 = call-dynamic "Start Lock-In Channel.vi"("instance"=0 ("index"), "error in"=w247, "config"=w240, "lia host in"=w245) -> ("error out"=w246:errorcluster, "lia host out"=w244:refnum<class "LIA Host Interface.lvclass">)  [unwired: 6 in]
          }
          event "lock-in.manual carrier 0": Value Change {
            n88 = event-data() -> ("NewVal"=w252:dbl)  [unwired: 1 in]
            n89 = expression code="-x/100000000"(w252) -> (w263:dbl)
            n90 = Bundle By Name(cluster=cluster{"config":T3, "record length":u32} {"config"={"decimation"=0, "source"=0, "carrier source"=0, "carrier"=0.0}, "record length"=0} ("config"), "record length"=w254, "config.source"=w251, "config.carrier source"=w262, "config.carrier"=w263, "config.decimation"=w261) -> (w253:cluster{"config":T3, "record length":u32})
            n91 = call-dynamic "Start Lock-In Channel.vi"("instance"=0 ("index"), "error in"=w260, "config"=w253, "lia host in"=w258) -> ("error out"=w259:errorcluster, "lia host out"=w257:refnum<class "LIA Host Interface.lvclass">)  [unwired: 6 in]
          }
          event "lock-in.boxcar length 0": Value Change {
            n92 = event-data() -> ("NewVal"=w265:u32)  [unwired: 1 in]
            n93 = expression code="-x/100000000"(w274) -> (w276:dbl)
            n94 = Bundle By Name(cluster=cluster{"config":T3, "record length":u32} {"config"={"decimation"=0, "source"=0, "carrier source"=0, "carrier"=0.0}, "record length"=0} ("config"), "record length"=w265, "config.source"=w264, "config.carrier source"=w275, "config.carrier"=w276, "config.decimation"=w273) -> (w266:cluster{"config":T3, "record length":u32})
            n95 = call-dynamic "Start Lock-In Channel.vi"("instance"=0 ("index"), "error in"=w272, "config"=w266, "lia host in"=w270) -> ("error out"=w271:errorcluster, "lia host out"=w269:refnum<class "LIA Host Interface.lvclass">)  [unwired: 6 in]
          }
          event "lock-in.decimation 0": Value Change {
            n96 = event-data() -> ("NewVal"=w281:i32)  [unwired: 1 in]
            n97 = expression code="-x/100000000"(w287) -> (w289:dbl)
            n98 = Bundle By Name(cluster=cluster{"config":T3, "record length":u32} {"config"={"decimation"=0, "source"=0, "carrier source"=0, "carrier"=0.0}, "record length"=0} ("config"), "record length"=w278, "config.source"=w280, "config.carrier source"=w288, "config.carrier"=w289, "config.decimation"=w281) -> (w277:cluster{"config":T3, "record length":u32})
            n99 = call-dynamic "Start Lock-In Channel.vi"("instance"=0 ("index"), "error in"=w286, "config"=w277, "lia host in"=w284) -> ("error out"=w285:errorcluster, "lia host out"=w283:refnum<class "LIA Host Interface.lvclass">)  [unwired: 6 in]
          }
          event "pll.q frequency 0": Value Change {
            n100 = event-data() -> ("NewVal"=w296:dbl)  [unwired: 1 in]
            n101 = expression code="x/100000000"(w296) -> (w299:dbl)
            n102 = Bundle By Name(cluster=T4 {"source"=0, "q frequency"=0.0} ("config"), "source"=w297, "q frequency"=w299) -> (w291:T4)
            n103 = call-dynamic "Configure PLL.vi"("instance"=0, "error in"=w295, "config"=w291, "lia host in"=w294) -> ("error out"=w292:errorcluster, "lia host out"=w293:refnum<class "LIA Host Interface.lvclass">)  [unwired: 6 in]
          }
          event "lock-in.reset boxar 0": Value Change {
            n104 = event-data() -> ()  [unwired: 1 in, 1 out]
            n105 = property on="Result" class="WFChart (strict)"(error in=w303, "History Data"=cluster{"mean":dbl, "trace":dbl}[] []) -> (error out=w302:errorcluster)  [unwired: 1 in, 1 out]
          }
          event "ao.noise 3": Value Change {
            n106 = event-data() -> ("NewVal"=w304:dbl)  [unwired: 1 in]
            n107 = call-dynamic "Configure Noise Level.vi"("error in"=w307, "level"=w304, "lia host in"=w308) -> ("error out"=w305:errorcluster, "lia host out"=w306:refnum<class "LIA Host Interface.lvclass">)  [unwired: 7 in]
          }
        }
      }
      frame True {
      }
    }
    n108 = Or(x=w94, y=w95) -> (x .or. y?=w111:bool)
  }
  n109 = Send Notification(notification=TRUE, notifier=w31) -> (notifier out=w29:refnum<notifier>)  [unwired: 1 in, 1 out]
  n110 = Send Notification(notification=TRUE, notifier=w34) -> (notifier out=w30:refnum<notifier>)  [unwired: 1 in, 1 out]
  n111 = flat-sequence {
    tunnel: w30 -> [w313]
    tunnel: w29 -> [_]
    frame #0 {
      n112 = Release Notifier(notifier=w313) -> ()  [unwired: 2 in, 3 out]
    }
  }
  n113 = Merge Errors(w27, w28) -> (w26:errorcluster)
  n114 = call-dynamic "Close.vi"("error in"=w26, "lia host in"=w39) -> ("error out"=w2:errorcluster)  [unwired: 8 in, 1 out]
  n115 = call <vilib>:"Simple Error Handler.vi"("error in (no error)"=w2) -> ()  [unwired: 4 in, 5 out]
